vi "Cross Calibration.vi"(4 "RF data Out":T2={"Sampling Rate"=10, "Delay (micro s)"=0.08, "rf points per line"=3000} {"Delay (micro s)" format="%.2f"}, 6 "Vert Settings":cluster{u16, i32, "Coupling":u16}={4, 0, "Coupling"=2}, 8 "Motion Bd ID":T1=1 min=1 max=32 step=1) -> ()   [LabVIEW 2022 SP3]
uses:
  <instrlib>/Acqiris Dx/Acqiris Dx.lvlib
  ScanningControl/Motion Controllers/-MotionRoutines/MotionGlobals.vi
  <instrlib>/niScope/Acquire/Fetch/niScope Fetch.vi
  <vilib>/Utility/file.llb/Write To Spreadsheet File (string).vi
  <vilib>/Utility/file.llb/Write To Spreadsheet File (DBL).vi
  <vilib>/measure/NI_MAPro.lvlib
  <vilib>/measure/mascope.llb/Amplitude and Levels 1 chan.vi
  <vilib>/Math Plots/3D Math Plots/3D Surface/3D Surface Datatype/3D Surface Datatype.lvclass
  <vilib>/Math Plots/3D Math Plots/3D Surface/3D Surface Datatype/Public/Plot Helper (Vector).vi
  <vilib>/Analysis/NI_AALBase.lvlib
  <vilib>/Analysis/baseanly.llb/Mean (DBL).vi
  <vilib>/Math Plots/3D Math Plots/3D Surface/3D Surface XCtrl/3D Surface.xctl
panel:
  in  "Inverting Hydrophone?":bool
  in  "Main Digitizer":u16(ring)=1 items=["Acqiris Digitzer", "NI Digitizer"]
  in  "Notes":string="Tabor-DC Block-LPF-20dB attn- DC Block-ENI-Diode Expanders-PI50 ----- F22-06T-FOH System- Acqiris"
  in  "Amplifier Info":string="ENI 350L No Gauge"
  in  "Record Window (uS)":dbl=1.0
  in  "File Path":path=path "E:/Temp/PI50"
  in  "Auto Save Data?":bool
  out "Numeric":i32=8
  out "Numeric 2":i32=15
  in  "Save Waveforms":bool
  out "Waveform Array":dbl[][][](array[numeric])
  in  "Hydrophone Info":string="F22-06T"
  in  "Transducer Info":string(combo)="PI50-2-LPF-20dB"
  out "Ch 1":refnum<class "3D Plot Datatype.lvclass">[](xcontrol)
  out "Ch 0":refnum<class "3D Plot Datatype.lvclass">[](xcontrol)
  out "Ch 1":dbl[](graph)
  out "Ch 0":dbl[](graph)=[0.0, -0.000390625, -0.001953125, -0.0027343750000000003, -0.003125, -0.003125, -0.00390625, -0.004687500000000001, -0.005078125, -0.004687500000000001, -0.0027343750000000003, -0.00078125, 0.0015625, 0.0023437500000000003, 0.003515625, 0.004687500000000001, 0.005859375, 0.0054687500000000005, 0.004687500000000001, 0.00390625, 0.0027343750000000003, 0.000390625, -0.0027343750000000003, -0.004687500000000001, -0.005859375, -0.00625, -0.005859375, -0.00390625, -0.0023437500000000003, -0.000390625, 0.00078125, 0.0011718750000000002, 0.00078125, 0.0, -0.0015625, -0.0027343750000000003, -0.003515625, -0.00390625, -0.004296875, -0.0054687500000000005, -0.005859375, -0.0054687500000000005, -0.004687500000000001, -0.004296875, -0.00390625, -0.001953125, 0.00078125, 0.003515625, 0.003515625, 0.0027343750000000003, 0.00078125, -0.000390625, -0.0015625, -0.00078125, -0.00078125, -0.001953125, -0.00390625, -0.0054687500000000005, -0.00625, -0.005078125, -0.004687500000000001, -0.004296875, -0.003515625, -0.0015625, 0.000390625, 0.0015625, 0.0011718750000000002, 0.00078125, 0.0015625, 0.0027343750000000003, 0.0023437500000000003, 0.0, -0.0015625, -0.001953125, -0.00078125, -0.000390625, -0.000390625, 0.0, 0.000390625, 0.0011718750000000002, 0.0023437500000000003, 0.00390625, 0.004296875, 0.004687500000000001, 0.005078125, 0.005859375, 0.0054687500000000005, 0.004687500000000001, 0.003125, 0.001953125, 0.0, -0.001953125, -0.004296875, -0.00625, -0.00703125, -0.00703125, -0.004687500000000001, -0.003125, -0.0015625, -0.000390625, 0.000390625, 0.0, -0.0011718750000000002, -0.0027343750000000003, -0.004296875, -0.005078125, -0.005078125, -0.005859375, -0.00625, -0.006640625000000001, -0.00625, -0.00390625, -0.001953125, -0.0015625, -0.0011718750000000002, 0.0011718750000000002, 0.0023437500000000003, 0.003125, 0.003125, 0.003125, 0.003515625, 0.003125, 0.0027343750000000003, 0.0011718750000000002, -0.0015625, -0.003125, -0.003515625, -0.0011718750000000002, 0.0015625, 0.004687500000000001, 0.005859375, 0.0054687500000000005, 0.004296875, 0.003125, 0.0023437500000000003, 0.000390625, -0.0011718750000000002, -0.0023437500000000003, -0.003515625, -0.004687500000000001, -0.005078125, -0.005859375, -0.006640625000000001, -0.00703125, -0.0054687500000000005, -0.0027343750000000003, -0.000390625, 0.00078125, 0.0011718750000000002, 0.0015625, 0.0015625, 0.003515625, 0.003515625, 0.0015625, -0.00078125, -0.0015625, -0.001953125, -0.0015625, -0.0015625, -0.001953125, -0.001953125, -0.00078125, 0.00078125, 0.003125, 0.00390625, 0.00390625, 0.003125, 0.0027343750000000003, 0.0027343750000000003, 0.0023437500000000003, 0.0027343750000000003, 0.0011718750000000002, -0.00078125, -0.0027343750000000003, -0.0027343750000000003, -0.0023437500000000003, -0.0015625, -0.001953125, -0.003125, -0.003125, -0.0027343750000000003, -0.0011718750000000002, 0.0, 0.00078125, -0.00078125, -0.0015625, -0.0023437500000000003, -0.0027343750000000003, -0.00390625, -0.0054687500000000005, -0.005859375, -0.004687500000000001, -0.0027343750000000003, -0.0015625, -0.0015625, -0.000390625, -0.000390625, 0.00078125, 0.001953125, 0.0023437500000000003, 0.0027343750000000003, 0.0015625, 0.0, -0.0011718750000000002, -0.0015625, -0.001953125, -0.001953125, -0.001953125, -0.001953125, -0.00078125, -0.000390625, -0.000390625, 0.0, 0.0015625, 0.00390625, 0.0054687500000000005, 0.005859375, 0.0054687500000000005, 0.004687500000000001, 0.0027343750000000003, 0.00078125, -0.0011718750000000002, -0.003125, -0.0027343750000000003, -0.0027343750000000003, -0.0023437500000000003, -0.003515625, -0.003515625, -0.003515625, -0.0027343750000000003, -0.0015625, -0.00078125, -0.00078125, -0.0015625, -0.0023437500000000003, -0.0027343750000000003, -0.003515625, -0.00390625, -0.00390625, -0.005078125, -0.00703125, -0.0078125, -0.00703125, -0.0054687500000000005, -0.003125, -0.001953125, -0.00078125, 0.0, 0.000390625, 0.0, -0.0011718750000000002, -0.0023437500000000003, -0.00390625, -0.004687500000000001, -0.005078125, -0.005078125, -0.0054687500000000005, -0.006640625000000001, -0.006640625000000001, -0.00625, -0.004687500000000001, -0.003515625, -0.003515625, -0.003125, -0.0023437500000000003, -0.000390625, 0.0011718750000000002, 0.00078125, -0.000390625, -0.001953125, -0.0023437500000000003, -0.003125, -0.003515625, -0.00390625, -0.004687500000000001, -0.004296875, -0.003515625, -0.0023437500000000003, -0.000390625, 0.00078125, 0.001953125, 0.00390625, 0.005078125, 0.0054687500000000005, 0.00390625, 0.003515625, 0.0023437500000000003, 0.00078125, -0.0015625, -0.003125, -0.003125, -0.00390625, -0.004687500000000001, -0.0054687500000000005, -0.004687500000000001, -0.0027343750000000003, 0.0, 0.0023437500000000003, 0.003515625, 0.003515625, 0.00390625, 0.00390625, 0.003515625, 0.00078125, -0.0023437500000000003, -0.003125, -0.003125, -0.003125, -0.0023437500000000003, -0.0015625, -0.0011718750000000002, 0.0, 0.000390625, 0.0011718750000000002, 0.0015625, 0.0023437500000000003, 0.003125, 0.00390625, 0.003515625, 0.0023437500000000003, 0.00078125, -0.000390625, -0.001953125, -0.003125, -0.003125, -0.0027343750000000003, -0.0015625, -0.000390625, 0.0, 0.00078125, 0.0027343750000000003, 0.004296875, 0.004296875, 0.0023437500000000003, 0.0023437500000000003, 0.003515625, 0.005078125, 0.004687500000000001, 0.0023437500000000003, 0.0, -0.000390625, 0.0011718750000000002, 0.003125, 0.003125, 0.0015625, 0.000390625, 0.00078125, 0.0027343750000000003, 0.004687500000000001, 0.005859375, 0.004687500000000001, 0.003515625, 0.003125, 0.0027343750000000003, 0.003125, 0.0023437500000000003, 0.000390625, -0.00078125, -0.00078125, -0.000390625, 0.0, 0.0, 0.00078125, 0.0027343750000000003, 0.004687500000000001, 0.005078125, 0.004687500000000001, 0.004687500000000001, 0.005078125, 0.005078125, 0.003515625, 0.00078125, -0.0015625, -0.0015625, -0.0015625, -0.0015625, -0.00078125, -0.000390625, 0.000390625, 0.0011718750000000002, 0.0015625, 0.001953125, 0.0027343750000000003, 0.003515625, 0.00390625, 0.004296875, 0.00390625, 0.0023437500000000003, 0.000390625, -0.0011718750000000002, -0.0015625, -0.0023437500000000003, -0.0027343750000000003, -0.003125, -0.001953125, 0.00078125, 0.0027343750000000003, 0.004687500000000001, 0.0054687500000000005, 0.005859375, 0.005078125, 0.004296875, 0.003515625, 0.001953125, -0.000390625, -0.003125, -0.005078125, -0.00625, -0.006640625000000001, -0.00625, -0.005859375, -0.004296875, -0.003125, -0.0023437500000000003, -0.0015625, -0.000390625, 0.00078125, 0.0015625, 0.0015625, 0.0015625, 0.000390625, -0.0015625, -0.0023437500000000003, -0.0023437500000000003, -0.0023437500000000003, -0.001953125, -0.001953125, -0.0015625, -0.00078125, 0.0, 0.00078125, 0.0015625, 0.00078125, -0.000390625, -0.0023437500000000003, -0.0027343750000000003, -0.001953125, -0.0023437500000000003, -0.003515625, -0.004296875, -0.004687500000000001, -0.004296875, -0.004687500000000001, -0.005078125, -0.004687500000000001, -0.003125, -0.0015625, -0.00078125, -0.000390625, 0.000390625, 0.0011718750000000002, 0.001953125, 0.0015625, 0.0015625, 0.0015625, 0.0011718750000000002, 0.00078125, 0.000390625, -0.000390625, -0.0015625, -0.0011718750000000002, 0.000390625, 0.0015625, 0.0027343750000000003, 0.003515625, 0.004296875, 0.004296875, 0.004296875, 0.004296875, 0.004296875, 0.0027343750000000003, 0.0011718750000000002, -0.000390625, -0.0011718750000000002, -0.0015625, -0.001953125, -0.0015625, -0.00078125, 0.0, 0.0015625, 0.003125, 0.004296875, 0.0054687500000000005, 0.005859375, 0.00625, 0.00625, 0.005078125, 0.003125, 0.0011718750000000002, -0.00078125, -0.001953125, -0.003515625, -0.0054687500000000005, -0.006640625000000001, -0.006640625000000001, -0.005078125, -0.004296875, -0.0027343750000000003, -0.0023437500000000003, -0.00078125, 0.00078125, 0.001953125, 0.0011718750000000002, -0.00078125, -0.0023437500000000003, -0.0023437500000000003, -0.0015625, -0.00078125, -0.00078125, 0.0, 0.00078125, 0.001953125, 0.0023437500000000003, 0.0027343750000000003, 0.0023437500000000003, 0.001953125, 0.0023437500000000003, 0.003515625, 0.003515625, 0.0023437500000000003, 0.0011718750000000002, 0.000390625, 0.00078125, 0.00078125, -0.00078125, -0.003125, -0.003515625, -0.0027343750000000003, -0.0011718750000000002, -0.000390625, -0.0011718750000000002, -0.001953125, -0.0015625, 0.0, 0.00078125, 0.000390625, -0.00078125, -0.0011718750000000002, -0.00078125, -0.00078125, -0.001953125, -0.004687500000000001, -0.005859375, -0.004687500000000001, -0.0023437500000000003, -0.00078125, 0.000390625, 0.0023437500000000003, 0.00390625, 0.004296875, 0.003515625, 0.0023437500000000003, 0.0027343750000000003, 0.003125, 0.003125, 0.001953125, 0.0011718750000000002, 0.0, -0.000390625, 0.0, 0.0011718750000000002, 0.001953125, 0.003125, 0.004296875, 0.0054687500000000005, 0.005859375, 0.00625, 0.006640625000000001, 0.00703125, 0.0054687500000000005, 0.003515625, 0.0011718750000000002, -0.00078125, -0.0011718750000000002, -0.001953125, -0.0015625, -0.001953125, -0.0011718750000000002, 0.00078125, 0.0027343750000000003, 0.004296875, 0.004296875, 0.00390625, 0.00390625, 0.003125, 0.003125, 0.0011718750000000002, -0.0015625, -0.00390625, -0.004687500000000001, -0.004687500000000001, -0.004296875, -0.004296875, -0.00390625, -0.003125, -0.0015625, -0.000390625, 0.0, 0.0, -0.000390625, -0.000390625, -0.000390625, -0.00078125, -0.001953125, -0.003125, -0.003515625, -0.003515625, -0.003125, -0.003515625, -0.003125, -0.0023437500000000003, -0.00078125, 0.0011718750000000002, 0.003125, 0.004687500000000001, 0.005859375, 0.00703125, 0.0078125, 0.005859375, 0.004296875, 0.003125, 0.0015625, 0.000390625, 0.0, -0.000390625, -0.0011718750000000002, -0.001953125, -0.0015625, -0.000390625, 0.0011718750000000002, 0.0011718750000000002, 0.0, -0.0027343750000000003, -0.003515625, -0.0023437500000000003, -0.0015625, -0.0015625, -0.0023437500000000003, -0.0023437500000000003, -0.003125, -0.00390625, -0.004687500000000001, -0.004687500000000001, -0.00390625, -0.003515625, -0.0023437500000000003, -0.0015625, 0.0, 0.0015625, 0.0027343750000000003, 0.004296875, 0.004687500000000001, 0.003515625, 0.0023437500000000003, 0.0015625, 0.00078125, 0.0, -0.0015625, -0.0015625, -0.000390625, 0.000390625, 0.000390625, -0.000390625, -0.00078125, -0.000390625, 0.00078125, 0.0015625, 0.0015625, 0.0015625, 0.000390625, -0.00078125, -0.001953125, -0.003125, -0.004296875, -0.004687500000000001, -0.005078125, -0.004296875, -0.0023437500000000003, 0.0, 0.0015625, 0.003125, 0.005078125, 0.006640625000000001, 0.0074218750000000005, 0.008203125, 0.0074218750000000005, 0.006640625000000001, 0.00390625, 0.00078125, -0.0023437500000000003, -0.003125, -0.0023437500000000003, -0.0015625, 0.0, 0.000390625, 0.00078125, 0.001953125, 0.005859375, 0.008203125, 0.0078125, 0.005859375, 0.00390625, 0.0027343750000000003, 0.0015625, -0.00078125, -0.003515625, -0.004687500000000001, -0.004296875, -0.004296875, -0.003515625, -0.0027343750000000003, 0.0, 0.001953125, 0.004296875, 0.004687500000000001, 0.003125, 0.003515625, 0.00390625, 0.004296875, 0.00390625, 0.003515625, 0.003125, 0.001953125, 0.000390625, -0.00078125, -0.0011718750000000002, -0.0015625, -0.00078125, 0.000390625, 0.00078125, 0.0015625, 0.00078125, 0.0011718750000000002, 0.0015625, 0.0023437500000000003, 0.001953125, 0.00078125, -0.0015625, -0.003515625, -0.004687500000000001, -0.005078125, -0.00625, -0.0078125, -0.008203125, -0.00625, -0.001953125, 0.0011718750000000002, 0.0027343750000000003, 0.003515625, 0.00390625, 0.003515625, 0.0027343750000000003, 0.00078125, -0.00078125, -0.0023437500000000003, -0.004296875, -0.006640625000000001, -0.0078125, -0.0074218750000000005, -0.004687500000000001, -0.0015625, 0.00078125, 0.00078125, 0.00078125, 0.0011718750000000002, 0.0015625, 0.001953125, 0.0015625, 0.0011718750000000002, 0.000390625, -0.0015625, -0.003125, -0.004687500000000001, -0.005078125, -0.00390625, -0.00078125, 0.0015625, 0.003125, 0.003125, 0.003125, 0.004296875, 0.0054687500000000005, 0.006640625000000001, 0.00703125, 0.006640625000000001, 0.005078125, 0.003515625, 0.0015625, 0.0, -0.00078125, -0.00078125, 0.0, -0.00078125, -0.00078125, 0.0, 0.001953125, 0.003125, 0.00390625, 0.004687500000000001, 0.004296875, 0.0027343750000000003, 0.0, -0.0023437500000000003, -0.003515625, -0.00390625, -0.003125, -0.0027343750000000003, -0.0027343750000000003, -0.003125, -0.003125, -0.0027343750000000003, -0.0023437500000000003, -0.0023437500000000003, -0.0027343750000000003, -0.0023437500000000003, -0.0015625, -0.000390625, 0.000390625, 0.000390625, -0.000390625, -0.0015625, -0.0023437500000000003, -0.0015625, -0.000390625, 0.0, 0.00078125, 0.0023437500000000003, 0.004687500000000001, 0.005859375, 0.005859375, 0.004687500000000001, 0.004296875, 0.003515625, 0.0023437500000000003, 0.0015625, 0.000390625, -0.000390625, -0.0015625, -0.0023437500000000003, -0.003515625, -0.00390625, -0.0023437500000000003, -0.00078125, 0.00078125, 0.000390625, 0.000390625, 0.0011718750000000002, 0.003125, 0.004687500000000001, 0.005078125, 0.004296875, 0.00390625, 0.004296875, 0.00390625, 0.0027343750000000003, 0.0015625, 0.00078125, 0.0, -0.00078125, -0.00078125, 0.000390625, 0.0015625, 0.003125, 0.004296875, 0.004687500000000001, 0.005078125, 0.00625, 0.006640625000000001, 0.0054687500000000005, 0.004296875, 0.0023437500000000003, 0.001953125, 0.001953125, 0.0027343750000000003, 0.001953125, 0.0, -0.0015625, -0.001953125, -0.0015625, -0.000390625, 0.00078125, 0.0011718750000000002, 0.0011718750000000002, -0.000390625, -0.0015625, -0.0027343750000000003, -0.0023437500000000003, -0.001953125, -0.0015625, -0.001953125, -0.003125, -0.00390625, -0.004296875, -0.004296875, -0.003125, -0.0015625, -0.000390625, 0.00078125, 0.003125, 0.005859375, 0.00703125, 0.00703125, 0.004687500000000001, 0.003125, 0.0015625, 0.000390625, -0.000390625, -0.000390625, -0.000390625, 0.0, 0.0011718750000000002, 0.0027343750000000003, 0.003515625, 0.00390625, 0.00390625, 0.004296875, 0.004687500000000001, 0.005078125, 0.0054687500000000005, 0.0054687500000000005, 0.004687500000000001, 0.003125, 0.0, -0.0023437500000000003, -0.001953125, 0.000390625, 0.0023437500000000003, 0.0023437500000000003, 0.0015625, 0.0011718750000000002, 0.0023437500000000003, 0.004687500000000001, 0.004687500000000001, 0.003515625, 0.0011718750000000002, -0.000390625, -0.00078125, 0.000390625, -0.00078125, -0.00390625, -0.00625, -0.006640625000000001, -0.006640625000000001, -0.005859375, -0.0054687500000000005, -0.004687500000000001, -0.003125, -0.000390625, 0.0023437500000000003, 0.00390625, 0.003125, 0.000390625, -0.0023437500000000003, -0.004687500000000001, -0.00390625, -0.0054687500000000005, -0.0078125, -0.008984375000000001, -0.00703125, -0.004296875, -0.0011718750000000002, 0.0015625, 0.0023437500000000003, 0.0027343750000000003, 0.004296875, 0.005859375, 0.006640625000000001, 0.005859375, 0.003515625, 0.0015625, 0.00078125, -0.000390625, -0.0015625, -0.0015625, -0.00078125, 0.000390625, 0.000390625, 0.0011718750000000002, 0.0023437500000000003, 0.003125, 0.00390625, 0.004296875, 0.00390625, 0.004296875, 0.004687500000000001, 0.003515625, 0.0023437500000000003, 0.0015625, 0.001953125, 0.001953125, 0.001953125, 0.0027343750000000003, 0.0023437500000000003, 0.0015625, 0.000390625, -0.0011718750000000002, 0.0, 0.0015625, 0.0027343750000000003, 0.004296875]
  out "Data Array":cluster{dbl[], dbl[], dbl[], dbl[]}={[30.0, 30.0, 30.0, 30.0, 30.0, 30.0, 30.0, 30.0, 30.0, 32.0, 32.0, 32.0, 32.0, 32.0, 32.0, 32.0, 32.0, 32.0, 34.0, 34.0, 34.0, 34.0, 34.0, 34.0, 34.0, 34.0, 34.0, 36.0, 36.0, 36.0, 36.0, 36.0, 36.0, 36.0, 36.0, 36.0, 38.0, 38.0, 38.0, 38.0, 38.0, 38.0, 38.0, 38.0, 38.0, 40.0, 40.0, 40.0, 40.0, 40.0, 40.0, 40.0, 40.0, 40.0, 42.0, 42.0, 42.0, 42.0, 42.0, 42.0, 42.0, 42.0, 42.0, 44.0, 44.0, 44.0, 44.0, 44.0, 44.0, 44.0, 44.0, 44.0, 46.0, 46.0, 46.0, 46.0, 46.0, 46.0, 46.0, 46.0, 46.0, 48.0, 48.0, 48.0, 48.0, 48.0, 48.0, 48.0, 48.0, 48.0, 50.0, 50.0, 50.0, 50.0, 50.0, 50.0, 50.0, 50.0, 50.0, 52.0, 52.0, 52.0, 52.0, 52.0, 52.0, 52.0, 52.0, 52.0, 54.0, 54.0, 54.0, 54.0, 54.0, 54.0, 54.0, 54.0, 54.0, 56.0, 56.0, 56.0, 56.0, 56.0, 56.0, 56.0, 56.0, 56.0, 58.0, 58.0, 58.0, 58.0, 58.0, 58.0, 58.0, 58.0, 58.0, 60.0, 60.0, 60.0, 60.0, 60.0, 60.0, 60.0, 60.0, 60.0], [0.1, 0.2, 0.30000000000000004, 0.4, 0.5, 0.6, 0.7000000000000001, 0.8, 0.9, 0.1, 0.2, 0.30000000000000004, 0.4, 0.5, 0.6, 0.7000000000000001, 0.8, 0.9, 0.1, 0.2, 0.30000000000000004, 0.4, 0.5, 0.6, 0.7000000000000001, 0.8, 0.9, 0.1, 0.2, 0.30000000000000004, 0.4, 0.5, 0.6, 0.7000000000000001, 0.8, 0.9, 0.1, 0.2, 0.30000000000000004, 0.4, 0.5, 0.6, 0.7000000000000001, 0.8, 0.9, 0.1, 0.2, 0.30000000000000004, 0.4, 0.5, 0.6, 0.7000000000000001, 0.8, 0.9, 0.1, 0.2, 0.30000000000000004, 0.4, 0.5, 0.6, 0.7000000000000001, 0.8, 0.9, 0.1, 0.2, 0.30000000000000004, 0.4, 0.5, 0.6, 0.7000000000000001, 0.8, 0.9, 0.1, 0.2, 0.30000000000000004, 0.4, 0.5, 0.6, 0.7000000000000001, 0.8, 0.9, 0.1, 0.2, 0.30000000000000004, 0.4, 0.5, 0.6, 0.7000000000000001, 0.8, 0.9, 0.1, 0.2, 0.30000000000000004, 0.4, 0.5, 0.6, 0.7000000000000001, 0.8, 0.9, 0.1, 0.2, 0.30000000000000004, 0.4, 0.5, 0.6, 0.7000000000000001, 0.8, 0.9, 0.1, 0.2, 0.30000000000000004, 0.4, 0.5, 0.6, 0.7000000000000001, 0.8, 0.9, 0.1, 0.2, 0.30000000000000004, 0.4, 0.5, 0.6, 0.7000000000000001, 0.8, 0.9, 0.1, 0.2, 0.30000000000000004, 0.4, 0.5, 0.6, 0.7000000000000001, 0.8, 0.9, 0.1, 0.2, 0.30000000000000004, 0.4, 0.5, 0.6, 0.7000000000000001, 0.8, 0.9], [0.004632148742675781, 0.012890625000000001, 0.02666015625, 0.040019531250000004, 0.05185546875, 0.059953498840332034, 0.06650390625, 0.07060546875, 0.0755859375, 0.004534759521484375, 0.012421875, 0.023457031250000003, 0.03400390625, 0.04359375, 0.05009765625, 0.05556640625, 0.059375, 0.063671875, 0.004769134521484375, 0.0134765625, 0.0256640625, 0.0360546875, 0.0433203125, 0.0474609375, 0.050820312500000006, 0.055703125000000006, 0.05859375, 0.005977287292480469, 0.014921875000000001, 0.02759765625, 0.03814453125, 0.04376953125, 0.0478515625, 0.052109375000000006, 0.0555859375, 0.0589453125, 0.005100135803222656, 0.01326171875, 0.02373046875, 0.0325, 0.0365234375, 0.039628906250000005, 0.04396484375, 0.046484375, 0.0507421875, 0.00481048583984375, 0.01208984375, 0.021328125000000003, 0.027714843750000002, 0.031542968750000004, 0.03357421875, 0.03666015625, 0.03853515625, 0.0409375, 0.0033821487426757813, 0.01138671875, 0.020722656250000002, 0.027246093750000002, 0.030507812500000002, 0.032207031250000004, 0.034824218750000004, 0.0376953125, 0.040156250000000004, 0.004744377136230469, 0.01, 0.01712890625, 0.020546875000000003, 0.02255859375, 0.024492187500000002, 0.025859375, 0.02880859375, 0.03125, 0.0044387817382812505, 0.008104858398437501, 0.01357421875, 0.015234375000000001, 0.01677734375, 0.01775390625, 0.0185546875, 0.019765625000000002, 0.021386718750000002, 0.004646453857421875, 0.007614898681640625, 0.0123828125, 0.014179687500000001, 0.01564453125, 0.0164453125, 0.017304687500000002, 0.0184765625, 0.0194921875, 0.00439453125, 0.0068927001953125, 0.011093750000000001, 0.01208984375, 0.01306640625, 0.01447265625, 0.015156250000000001, 0.0165234375, 0.01755859375, 0.00494110107421875, 0.004515190124511719, 0.010703125, 0.011484375, 0.01228515625, 0.0132421875, 0.01412109375, 0.015078125000000001, 0.016015625000000002, 0.003555717468261719, 0.006270446777343751, 0.00998046875, 0.01072265625, 0.01130859375, 0.012226562500000001, 0.01244140625, 0.0132421875, 0.014140625, 0.004312858581542969, 0.005177078247070313, 0.008241539001464845, 0.00966796875, 0.009765625, 0.010683593750000001, 0.011582031250000001, 0.012226562500000001, 0.0127734375, 0.004861183166503906, 0.005276260375976563, 0.007224807739257813, 0.006856727600097656, 0.008536224365234376, 0.008964920043945314, 0.010195312500000001, 0.010371093750000001, 0.0107421875, 0.005235977172851563, 0.004944725036621094, 0.00478424072265625, 0.0060133361816406255, 0.006972541809082032, 0.007910881042480469, 0.00812469482421875, 0.008906250000000001, 0.008612861633300781], [0.0, 0.0, 0.0, 0.0, 0.0, 0.0, 0.0, 0.0, 0.0, 0.0, 0.0, 0.0, 0.0, 0.0, 0.0, 0.0, 0.0, 0.0, 0.0, 0.0, 0.0, 0.0, 0.0, 0.0, 0.0, 0.0, 0.0, 0.0, 0.0, 0.0, 0.0, 0.0, 0.0, 0.0, 0.0, 0.0, 0.0, 0.0, 0.0, 0.0, 0.0, 0.0, 0.0, 0.0, 0.0, 0.0, 0.0, 0.0, 0.0, 0.0, 0.0, 0.0, 0.0, 0.0, 0.0, 0.0, 0.0, 0.0, 0.0, 0.0, 0.0, 0.0, 0.0, 0.0, 0.0, 0.0, 0.0, 0.0, 0.0, 0.0, 0.0, 0.0, 0.0, 0.0, 0.0, 0.0, 0.0, 0.0, 0.0, 0.0, 0.0, 0.0, 0.0, 0.0, 0.0, 0.0, 0.0, 0.0, 0.0, 0.0, 0.0, 0.0, 0.0, 0.0, 0.0, 0.0, 0.0, 0.0, 0.0, 0.0, 0.0, 0.0, 0.0, 0.0, 0.0, 0.0, 0.0, 0.0, 0.0, 0.0, 0.0, 0.0, 0.0, 0.0, 0.0, 0.0, 0.0, 0.0, 0.0, 0.0, 0.0, 0.0, 0.0, 0.0, 0.0, 0.0, 0.0, 0.0, 0.0, 0.0, 0.0, 0.0, 0.0, 0.0, 0.0, 0.0, 0.0, 0.0, 0.0, 0.0, 0.0, 0.0, 0.0, 0.0]}
  in  "Attenuator":dbl=1.0
  in  "Num Voltage Steps":i32=9
  in  "Average":i32=20
  out "current f":dbl=60.0
  in  "Freq Step Size (MHz)":dbl=2.0 format="%.2f"
  in  "Start frequency (MHz)":dbl=30.0 format="%.2f"
  in  "Cal Tran":bool
  in  "Set up Digi":bool
  in  "ExitSendCmd":bool
  in  "Save":bool
  out "current V":dbl=0.9
  in  "Function Generator":u16(ring)=1 items=["Agilent", "Tabor"]
  in  "Voltage Step Size (mVpp)":dbl=100.0 format="%.2f"
  in  "Num Freq Steps":i32=16
  in  "Start voltage (mVpp)":dbl=100.0 format="%.3f"
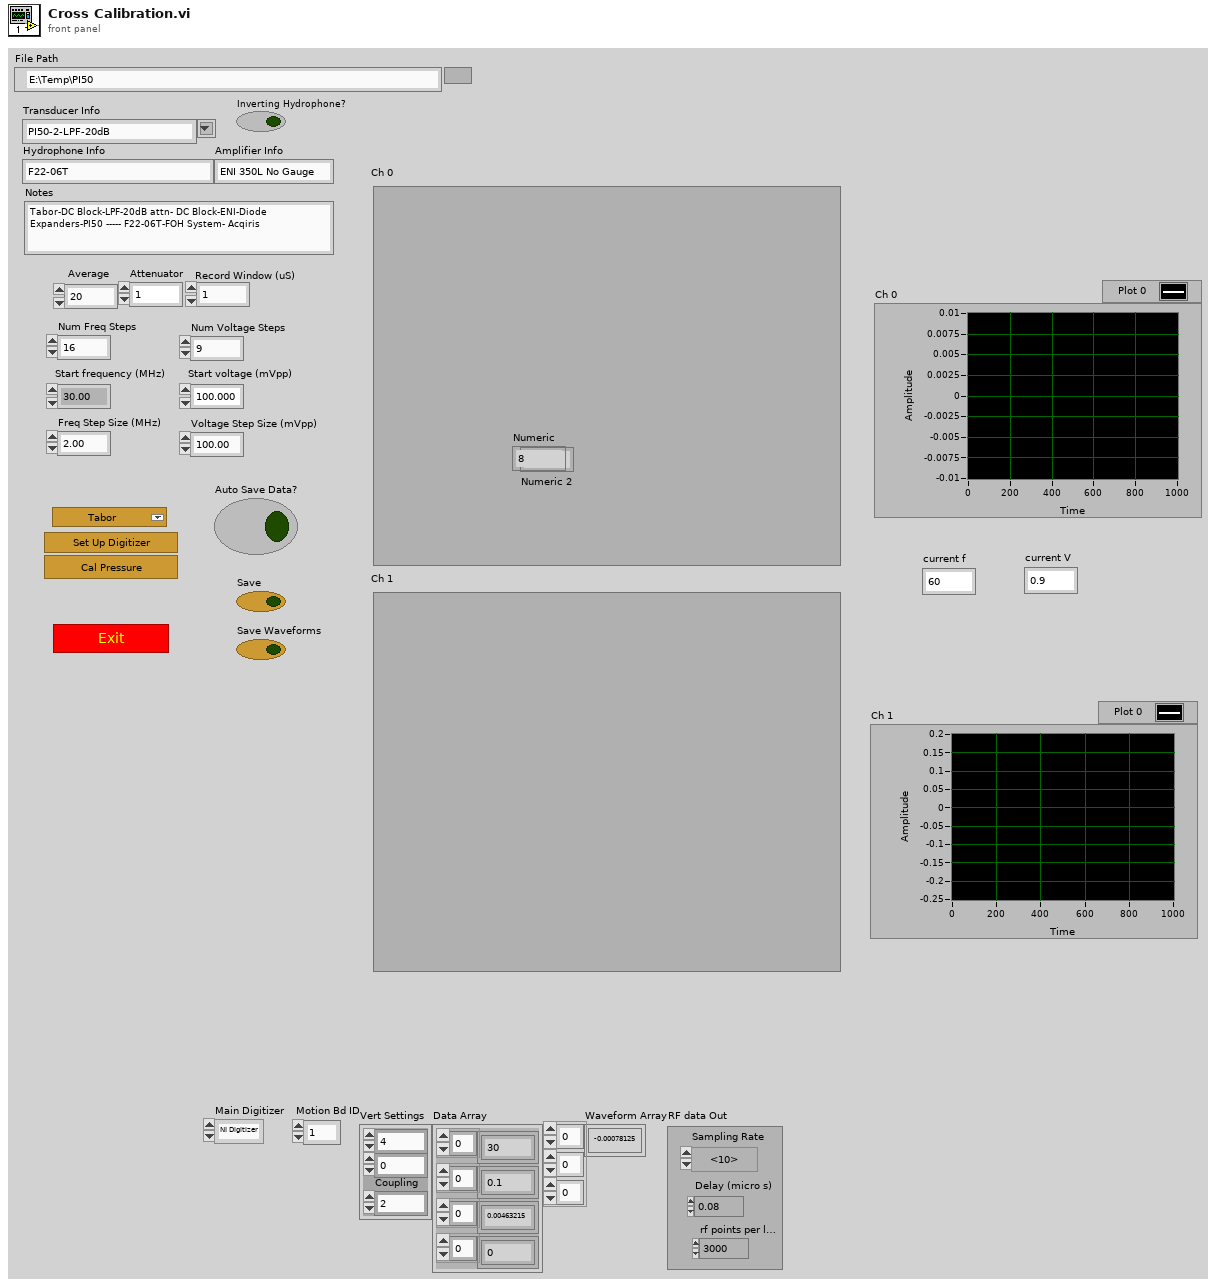
[diagram p1: front panel]
types:
  T1 = typedef "Board Id" = u8
  T2 = cluster{"Sampling Rate":u16, "Delay (micro s)":dbl, "rf points per line":u16}
  T3 = cluster{"Sampling Rate":dbl, "Ref Delay (ms)":dbl, "rf points per line":i32}
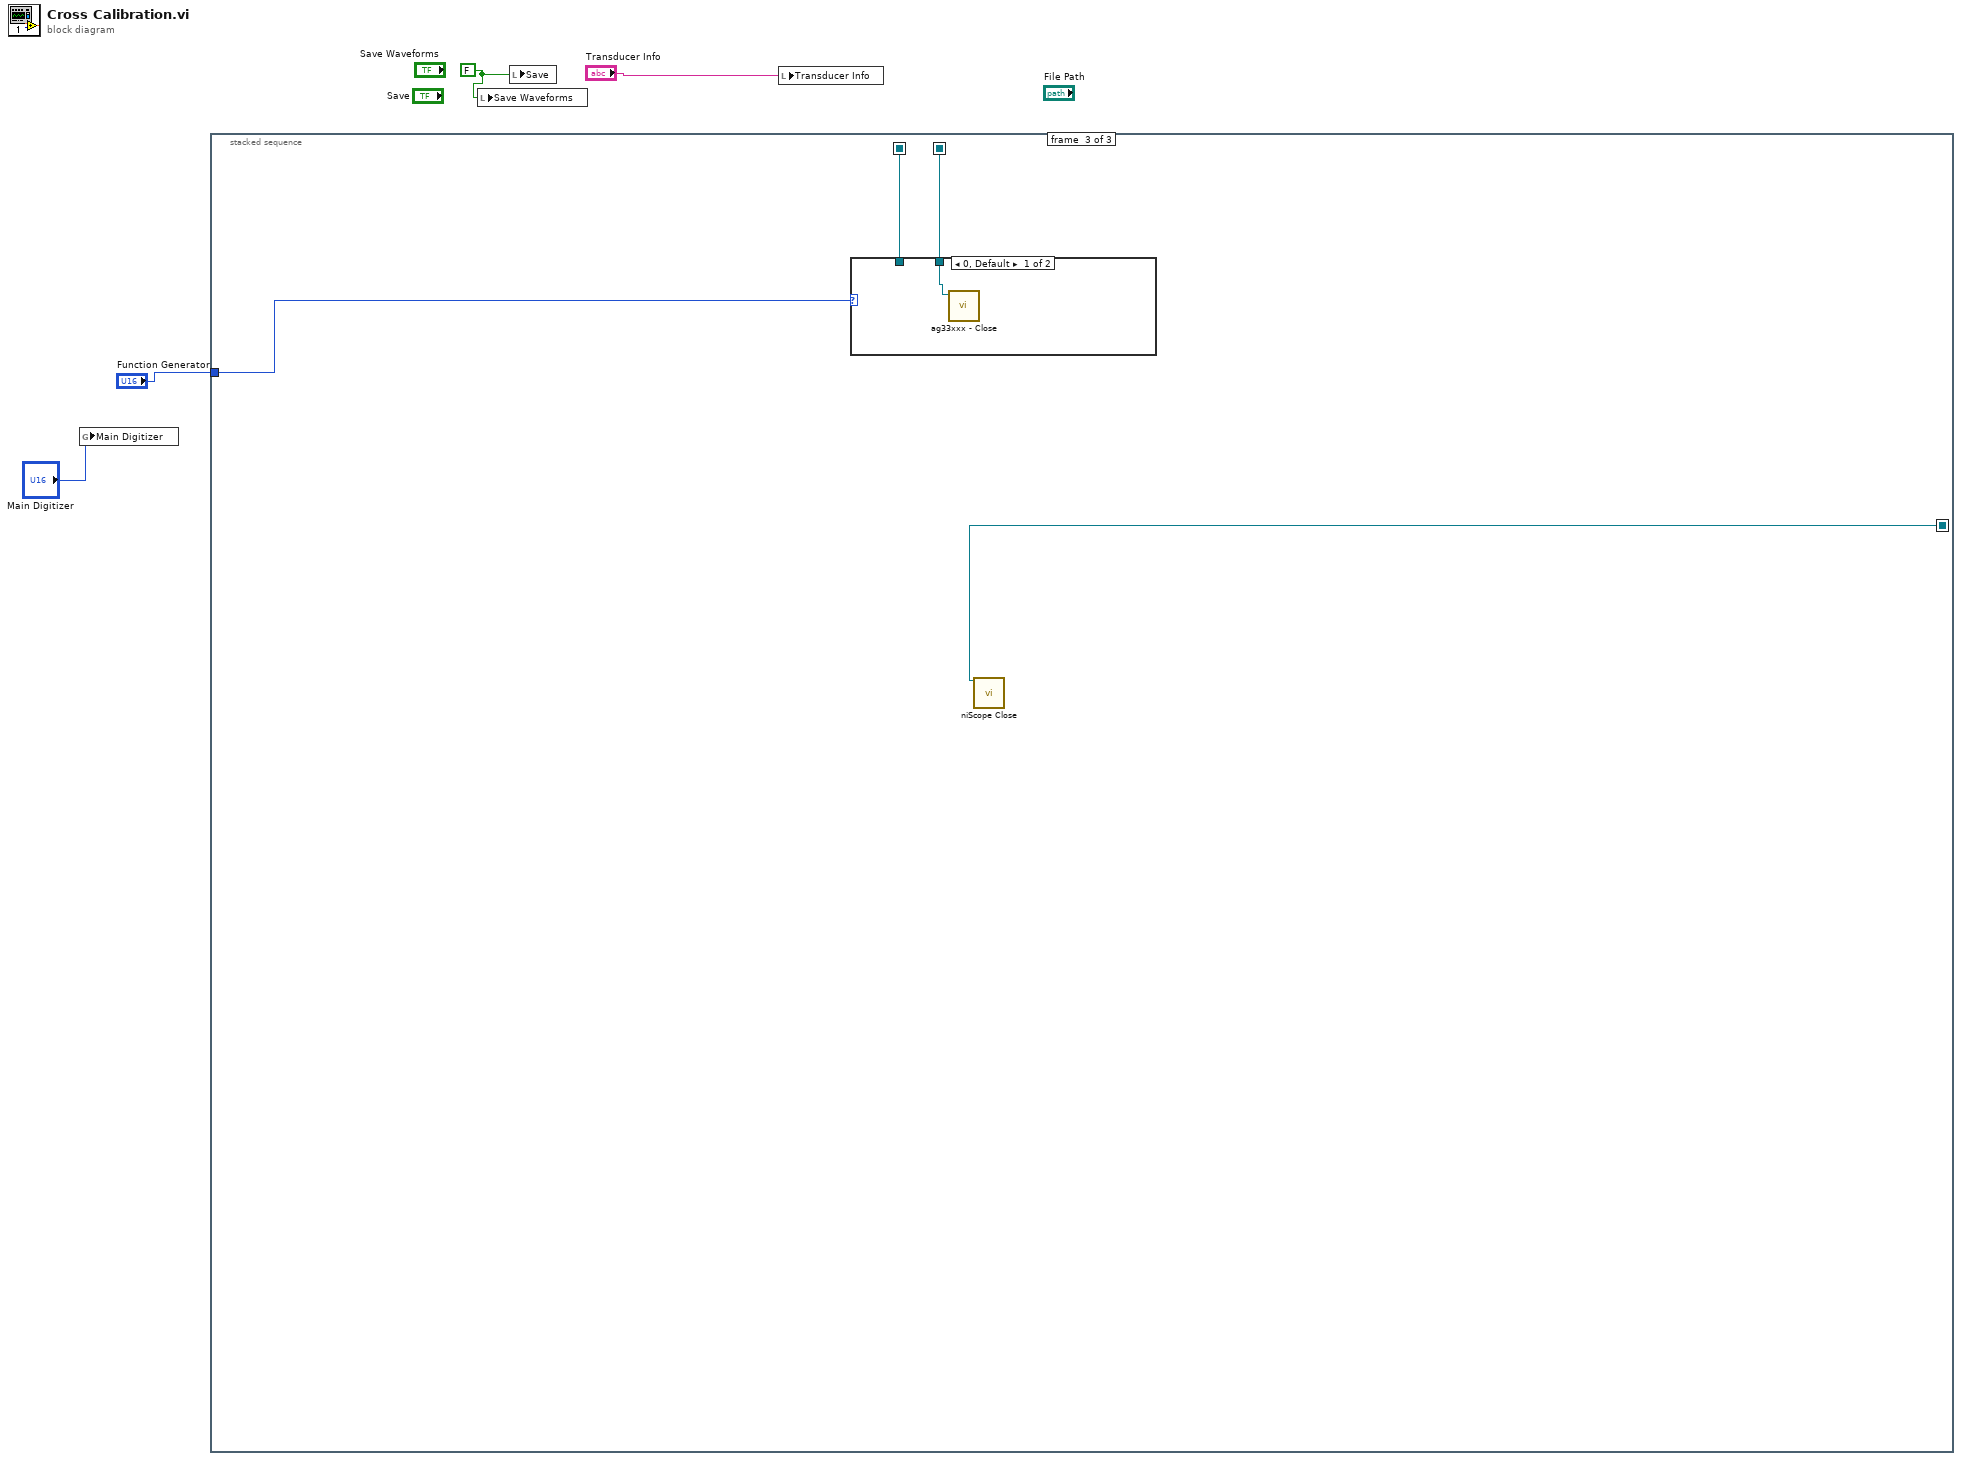
[diagram p0: block diagram]
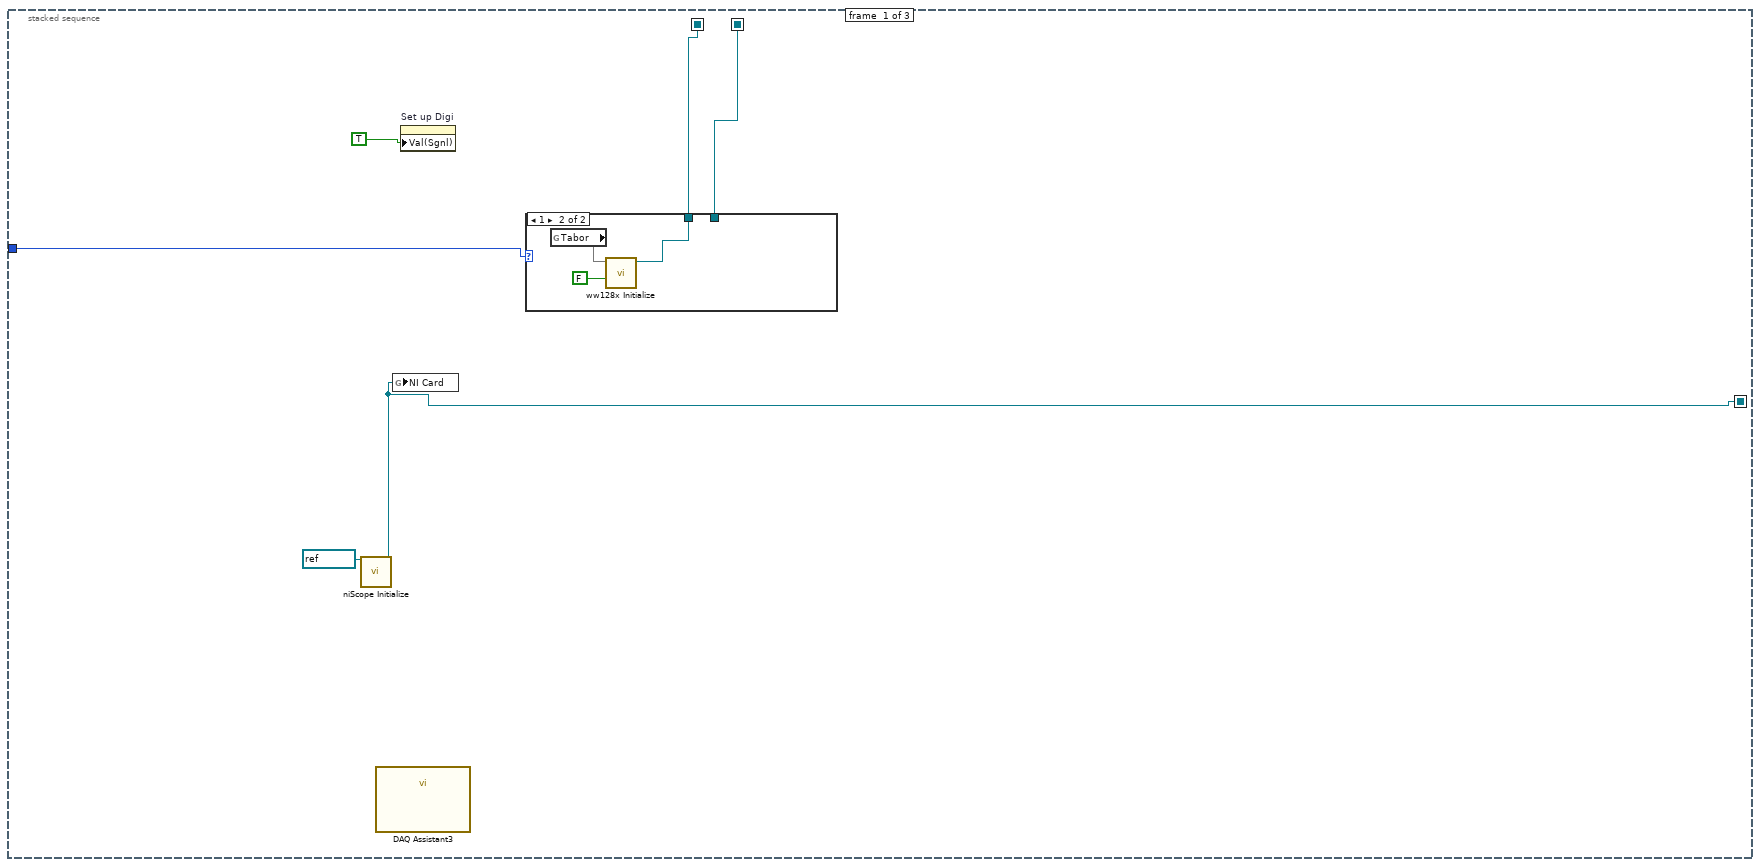
[diagram p2: hidden frame]
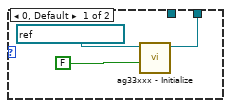
[diagram p3: hidden frame]
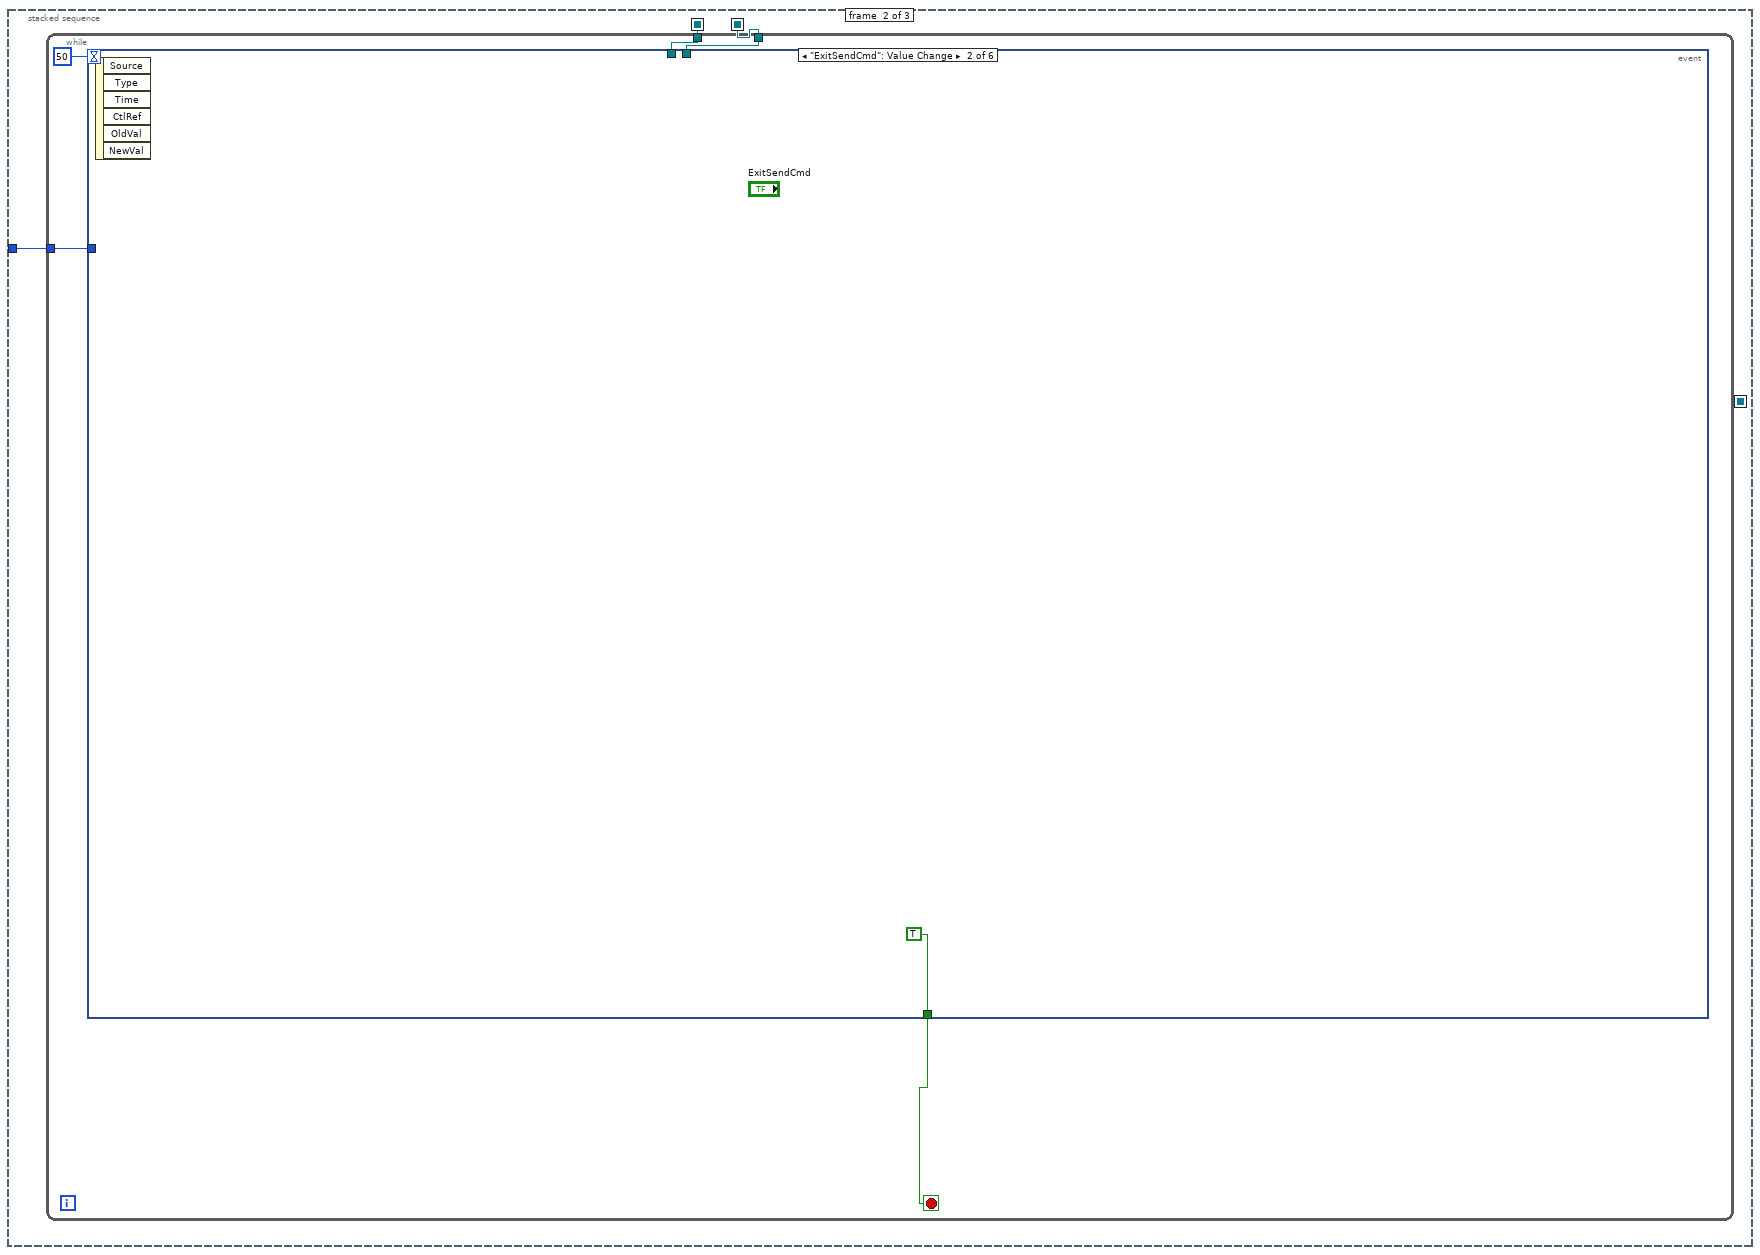
[diagram p4: hidden frame]
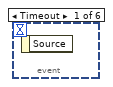
[diagram p5: hidden frame]
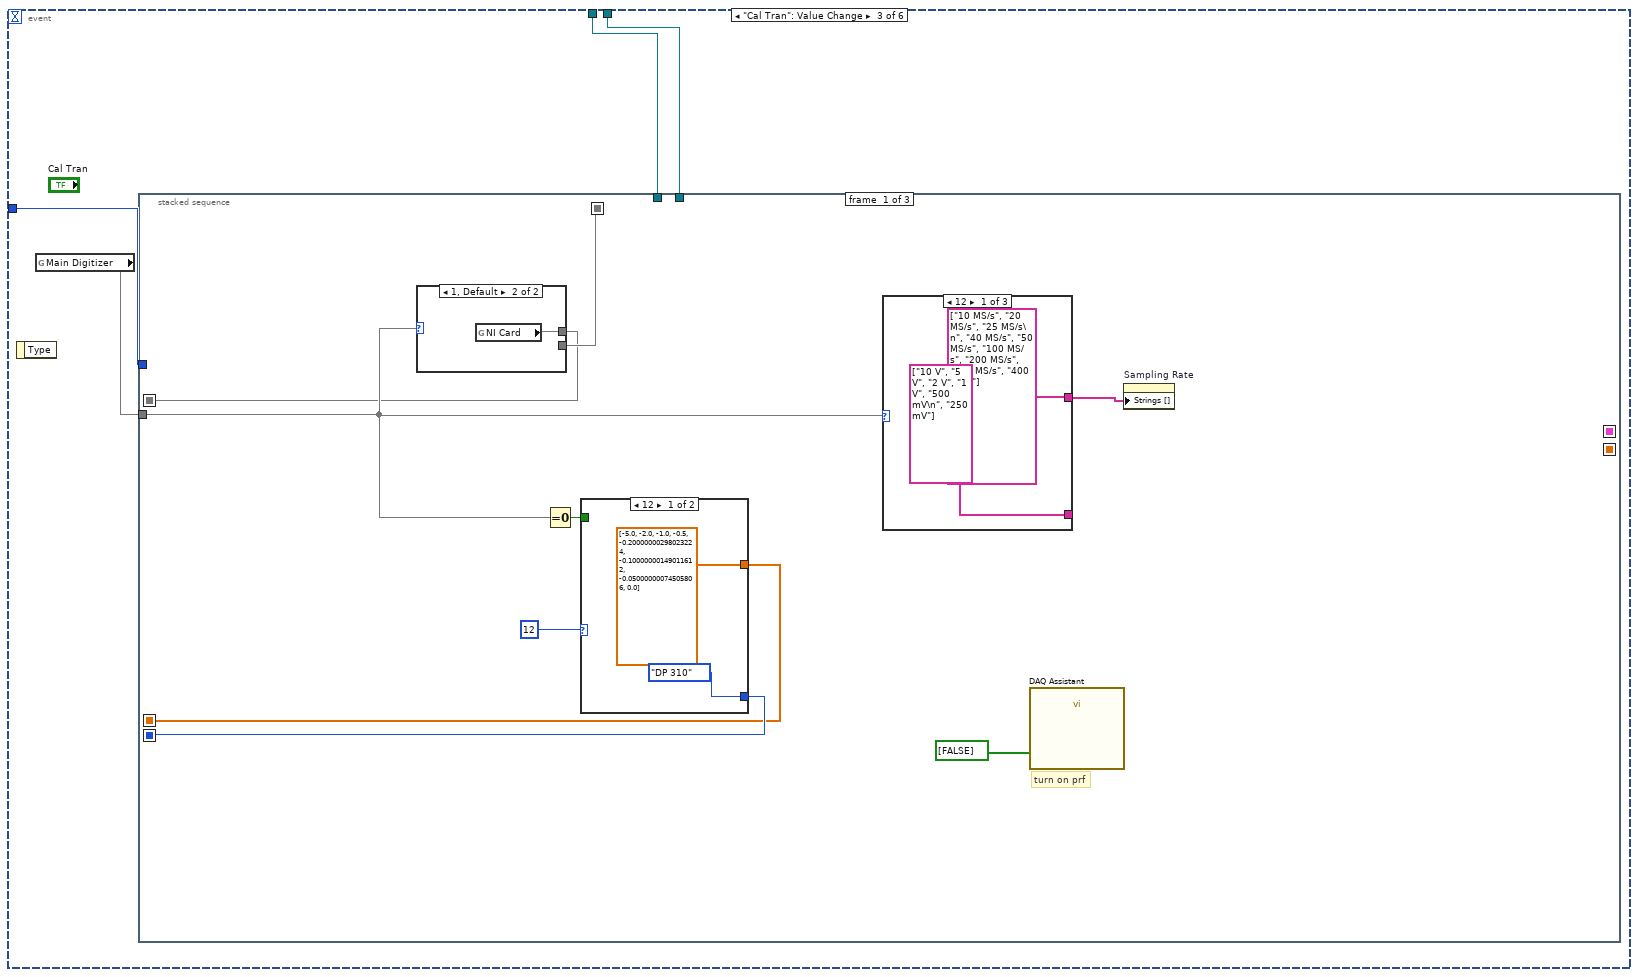
[diagram p6: hidden frame]
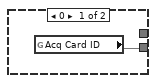
[diagram p7: hidden frame]
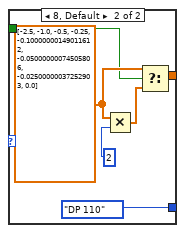
[diagram p8: hidden frame]
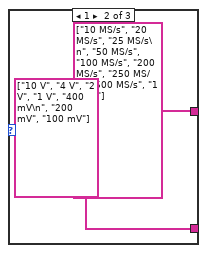
[diagram p9: hidden frame]
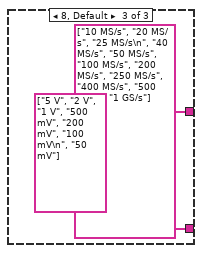
[diagram p10: hidden frame]
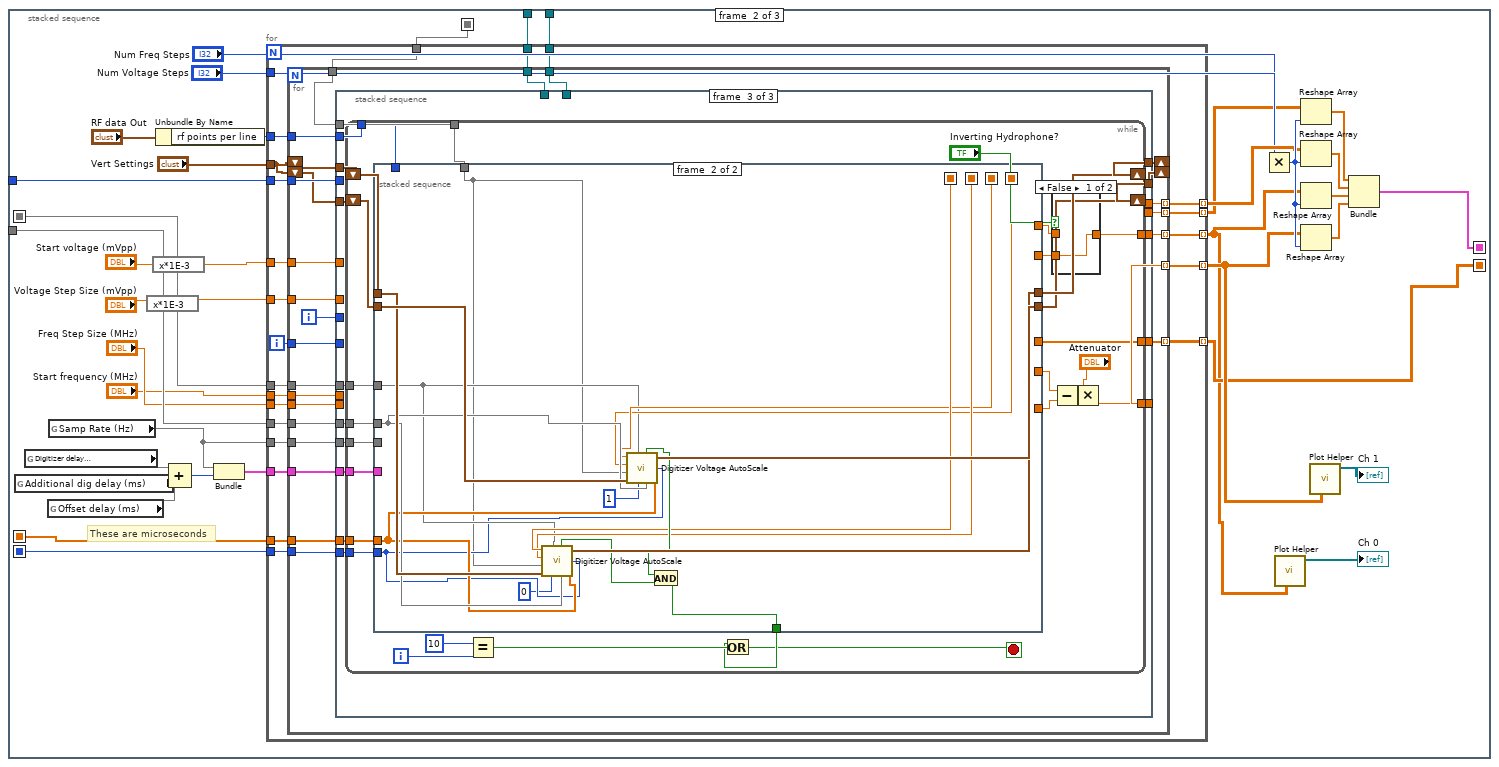
[diagram p11: hidden frame]
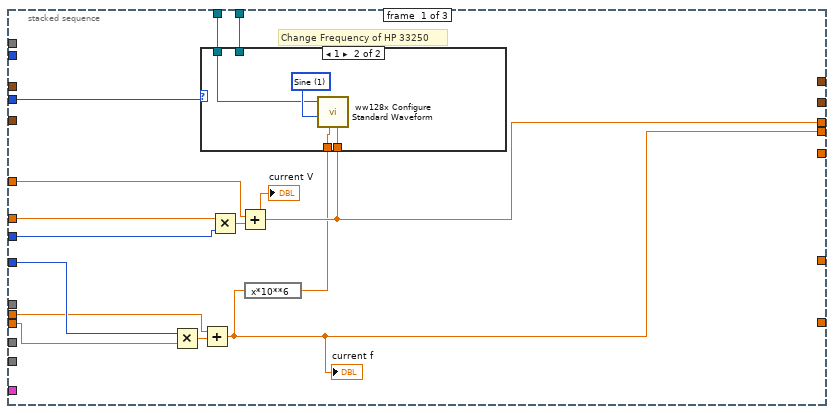
[diagram p12: hidden frame]
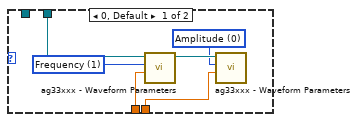
[diagram p13: hidden frame]
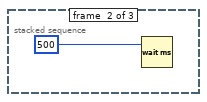
[diagram p14: hidden frame]
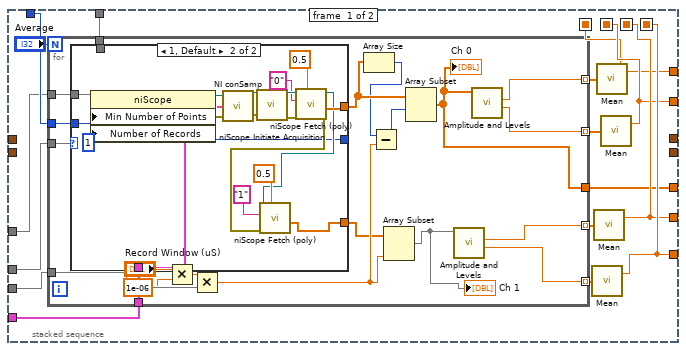
[diagram p16: hidden frame]
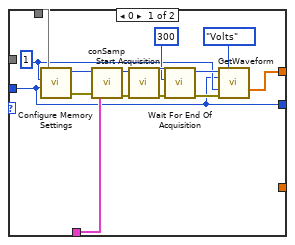
[diagram p17: hidden frame]
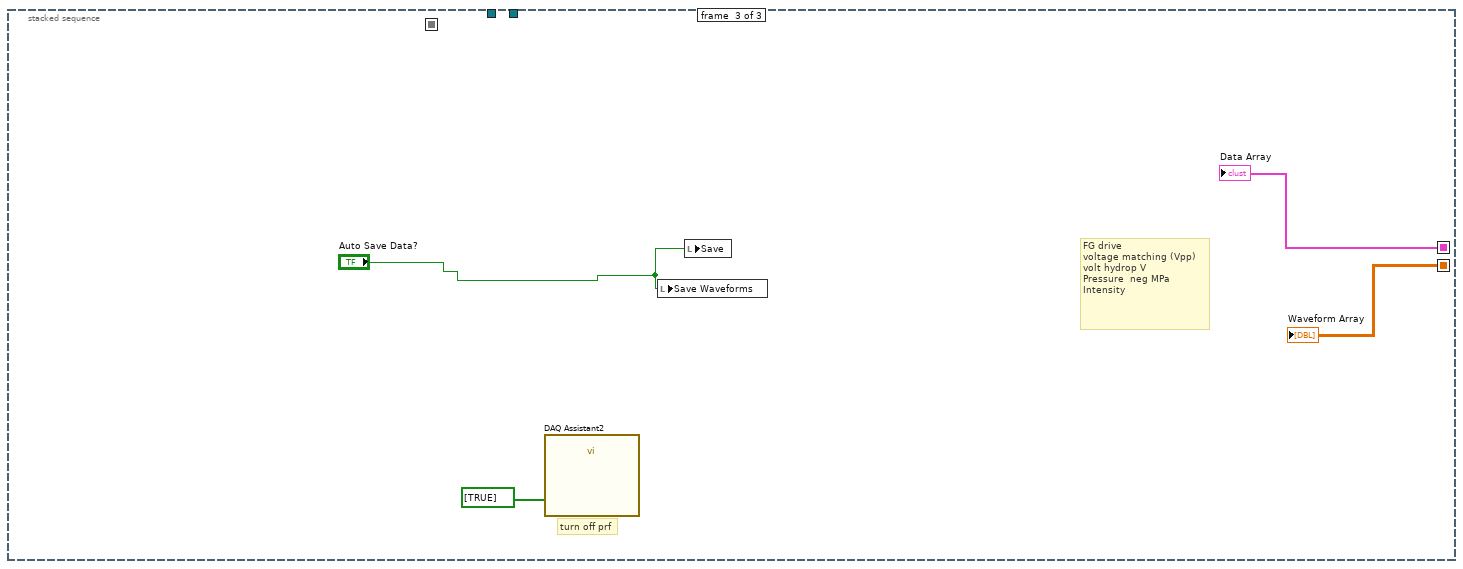
[diagram p18: hidden frame]
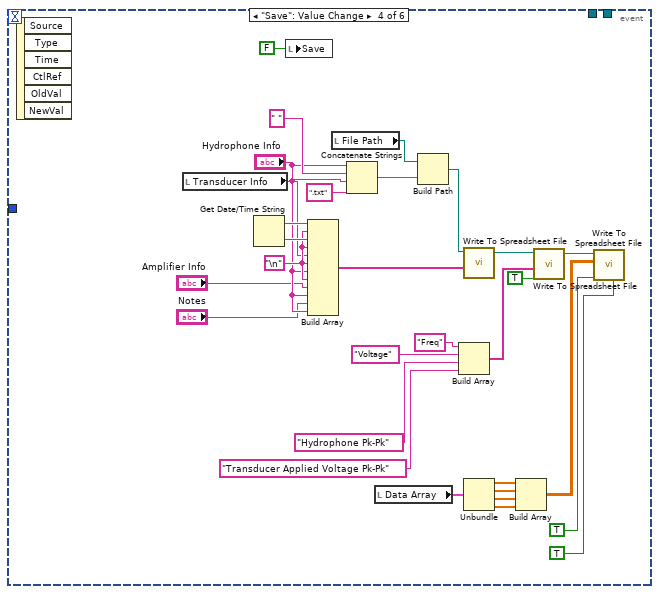
[diagram p19: hidden frame]
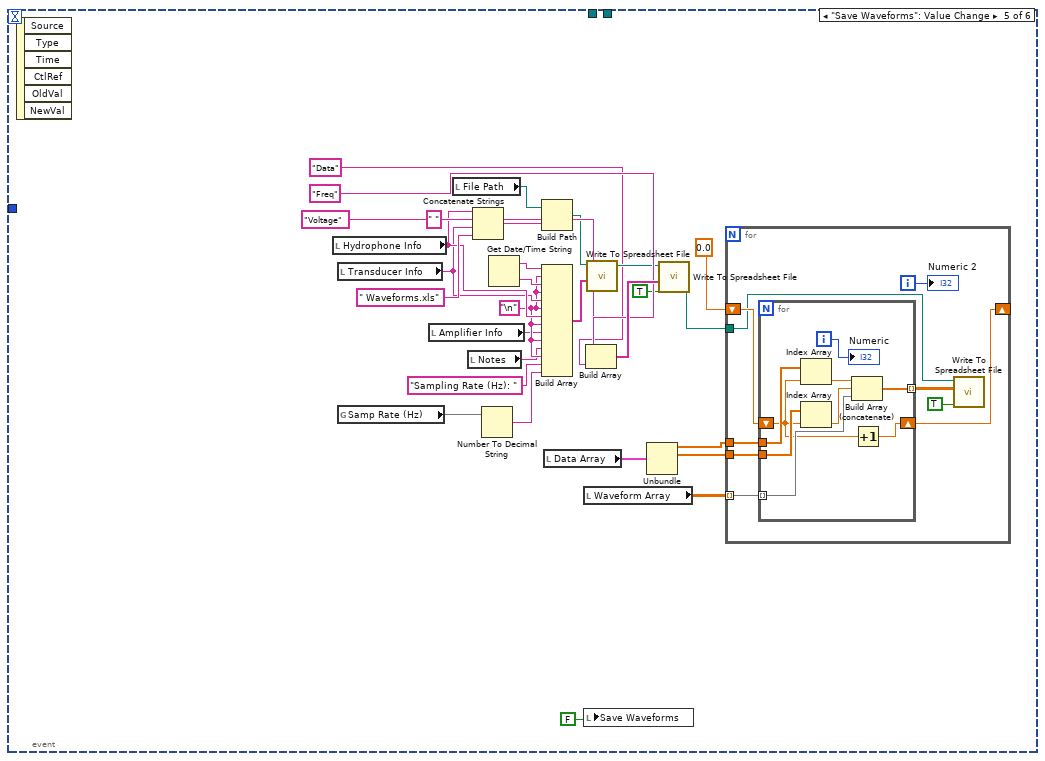
[diagram p20: hidden frame]
diagram:
  w1 = FALSE
  n1 = global write "MotionGlobals.vi" "Main Digitizer"("Main Digitizer") -> ()
  n2 = stacked-sequence {
    seq-local: [w8 _ _] -> [_ _ w388]
    seq-local: [w6 _ _] -> [_ w18 w386]
    seq-local: [w7 _ _] -> [_ w17 w385]
    tunnel: "Function Generator" -> [w9 w19 w387]
    frame #0 {
      n3 = call <instrlib>:"niScope Initialize.vi"("resource name"=refnum<k15> "DIG1") -> ("instrument handle"=w8:refnum<k15>)  [unwired: 3 in, 11 out]
      n4 = call "DAQ Assistant3"() -> ()  [unwired: 17 in, 3 out]
      n5 = global write "MotionGlobals.vi" "NI Card"(w8) -> ()
      n6 = property on="Set up Digi" class="Bool (strict)"("Val(Sgnl)"=TRUE) -> ()  [unwired: 2 in, 2 out]
      n7 = case shown="1" w9 {
        tunnel: [w12 _] -> w7
        tunnel: [_ w15] -> w6
        frame 0, Default {
          n8 = call <instrlib>:"ag33xxx - Initialize.vi"("Reset (T: Reset)"=FALSE, "Instrument Resource Name"=refnum<visa-resource-name> "GPIB::13::INSTR") -> ("dup VISA session"=w12:refnum<visa-resource-name>)  [unwired: 8 in, 1 out]
        }
        frame 1 {
          n9 = global read "MotionGlobals.vi" "Tabor"() -> (w14)
          n10 = call <instrlib>:"ww128x Initialize.vi"("reset device (Yes)"=FALSE ("reset device"), "resource name"=w14) -> ("instrument handle out"=w15:refnum<k15>)  [unwired: 2 in, 7 out]
        }
      }
    }
    frame #1 {
      n11 = while {
        tunnel: w19 -> [w22]
        tunnel: w18 -> [w21]
        tunnel: w17 -> [w20]
        stop <- w24 stop-if-true
        n12 = event shown="[1] \"ExitSendCmd\": Value Change" {
          selector: _ -> [_ _ _ _ _ _]
          dyn-events: _ -> [_ _ _ _ _ _]
          timeout: 50 -> [_ _ _ _ _ _]
          tunnel: [_ TRUE _ _ _ _] -> w24
          tunnel: w22 -> [_ _ w28 _ _ _]
          tunnel: w21 -> [_ _ w27 _ _ _]
          tunnel: w20 -> [_ _ w26 _ _ _]
          event Timeout {
            n13 = event-data() -> ()  [unwired: 2 out]
          }
          event "ExitSendCmd": Value Change {
            n14 = event-data() -> ()  [unwired: 7 out]
          }
          event "Cal Tran": Value Change {
            n15 = event-data() -> ()  [unwired: 2 out]
            n16 = global read "MotionGlobals.vi" "Main Digitizer"() -> (w29)
            n17 = stacked-sequence {
              seq-local: [w36 _ _] -> [_ w90 _]
              seq-local: [w37 _ _] -> [_ w91 _]
              seq-local: [w33 _ _] -> [_ w85 _]
              seq-local: [_ w76 _] -> [_ _ w300]
              seq-local: [w32 _ _] -> [_ w75 _]
              seq-local: [_ w57 _] -> [_ _ w299]
              tunnel: w29 -> [w35 w84 _]
              tunnel: w28 -> [_ w74 _]
              tunnel: w27 -> [_ w73 _]
              tunnel: w26 -> [_ w72 _]
              frame #0 {
                # "turn on prf"
                n18 = case shown="1, Default" w35 {
                  tunnel: [w39 _] -> w33
                  tunnel: [_ w40] -> w32
                  frame 0 {
                    n19 = global read "MotionGlobals.vi" "Acq Card ID"() -> (w39)
                  }
                  frame 1, Default {
                    n20 = global read "MotionGlobals.vi" "NI Card"() -> (w40)
                  }
                }
                n21 = Equal To 0?(x=w35) -> (x = 0?=w38:bool)
                n22 = case shown="12" 12 {
                  tunnel: [sgl[] [-5.0, -2.0, -1.0, -0.5, -0.2, -0.1, -0.05, 0.0] w43] -> w36
                  tunnel: [enum16{"DP 110", "DP 310"}."DP 310" ("Card Type") enum16{"DP 110", "DP 310"}."DP 110" ("Card Type")] -> w37
                  tunnel: w38 -> [_ w44]
                  frame 12 {
                  }
                  frame 8, Default {
                    w45 = sgl[] [-2.5, -1.0, -0.5, -0.25, -0.1, -0.05, -0.025, 0.0]
                    n23 = Multiply(x=w45, y=2) -> (x*y=w46:sgl[])
                    n24 = Select(t=w45, s=w44, f=w46) -> (s? t:f=w43:sgl[])
                  }
                }
                n25 = case shown="12" w35 {
                  tunnel: [string[] ["10 MS/s", "20 MS/s", "25 MS/s\n", "40 MS/s", "50 MS/s", "100 MS/s", "200 MS/s", "250 MS/s", "400 MS/s"] ("Strings []") string[] ["10 MS/s", "20 MS/s", "25 MS/s\n", "50 MS/s", "100 MS/s", "200 MS/s", "250 MS/s", "500 MS/s", "1 GS/s"] ("Strings []") string[] ["10 MS/s", "20 MS/s", "25 MS/s\n", "40 MS/s", "50 MS/s", "100 MS/s", "200 MS/s", "250 MS/s", "400 MS/s", "500 MS/s", "1 GS/s"] ("Strings []")] -> w34
                  tunnel: [string[] ["10 V", "5 V", "2 V", "1 V", "500 mV\n", "250 mV"] ("Strings []") string[] ["10 V", "4 V", "2 V", "1 V", "400 mV\n", "200 mV", "100 mV"] ("Strings []") string[] ["5 V", "2 V", "1 V", "500 mV", "200 mV", "100 mV\n", "50 mV"] ("Strings []")] -> _
                  frame 12 {
                  }
                  frame 1 {
                  }
                  frame 8, Default {
                  }
                }
                n26 = call "DAQ Assistant"("data"=bool[] [FALSE]) -> ()  [unwired: 3 in, 16 out]
                n27 = property on="Sampling Rate" class="Ring (strict)"("Strings []"=w34) -> ()  [unwired: 2 in, 2 out]
              }
              frame #1 {
                # "These are microseconds"
                n28 = global read "MotionGlobals.vi" "Additional dig delay (ms)"() -> (w82)
                n29 = global read "MotionGlobals.vi" "Digitizer delay\n (ms)"() -> (w80)
                n30 = global read "MotionGlobals.vi" "Offset delay (ms)"() -> (w83)
                n31 = global read "MotionGlobals.vi" "Samp Rate (Hz)"() -> (w68)
                n32 = expression code="x*1E-3"("Voltage Step Size (mVpp)") -> (w88:dbl)
                n33 = expression code="x*1E-3"("Start voltage (mVpp)") -> (w86:dbl)
                n34 = Unbundle By Name("RF data Out") -> ("rf points per line"=w92:u16)
                n35 = Compound Arithmetic op=ADD(w80, w82, w83) -> (w81:i32)
                n36 = Bundle("Samp Rate (Hz)"=w68, w81) -> (w79:cluster{"Samp Rate (Hz)":void, i32})  [unwired: 1 out]
                n37 = for {
                  N: "Num Freq Steps" -> [_]
                  tunnel: "Num Voltage Steps" -> [w115]
                  tunnel: w92 -> [w114]
                  tunnel: w91 -> [w113]
                  tunnel: w90 -> [w112]
                  tunnel: w88 -> [w111]
                  tunnel: w86 -> [w110]
                  tunnel: w85 -> [w109]
                  tunnel: w84 -> [w108]
                  tunnel: w79 -> [w107]
                  tunnel: "Vert Settings" -> [w95]
                  tunnel: w75 -> [w106]
                  tunnel: w74 -> [w105]
                  tunnel: w73 -> [w104]
                  tunnel: w72 -> [w103]
                  tunnel: "Freq Step Size (MHz)" -> [w101]
                  tunnel: "Start frequency (MHz)" -> [w100]
                  tunnel: w68 -> [w99]
                  tunnel: [w98] -> w55 mode=indexing
                  tunnel: [w97] -> w60 mode=indexing
                  tunnel: [w96] -> w56 mode=indexing
                  tunnel: [w93] -> w65 mode=indexing
                  tunnel: [w94] -> w57 mode=indexing
                  i -> [w102]
                  n38 = for {
                    N: w115 -> [_]
                    tunnel: w111 -> [w140]
                    tunnel: w110 -> [w139]
                    tunnel: w109 -> [w138]
                    tunnel: w114 -> [w137]
                    shift-right: [w136] -> _
                    shift-left: w95 -> [w135]
                    tunnel: w105 -> [w134]
                    tunnel: w112 -> [w133]
                    tunnel: w113 -> [w132]
                    tunnel: w108 -> [w131]
                    tunnel: w106 -> [w130]
                    tunnel: w107 -> [w129]
                    tunnel: w104 -> [w128]
                    tunnel: w103 -> [w127]
                    tunnel: w102 -> [w126]
                    tunnel: w101 -> [w125]
                    tunnel: w100 -> [w124]
                    tunnel: w99 -> [w123]
                    tunnel: [w122] -> w98 mode=indexing
                    tunnel: [w117] -> w97 mode=indexing
                    tunnel: [w121] -> w96 mode=indexing
                    tunnel: [w120] -> w93 mode=indexing
                    shift-right: [w119] -> _
                    shift-left: w95 -> [w118]
                    tunnel: [w116] -> w94 mode=indexing
                    i -> [w141]
                    n39 = stacked-sequence {
                      tunnel: w141 -> [w155 _ _]
                      tunnel: w140 -> [w154 _ _]
                      tunnel: w139 -> [w153 _ _]
                      tunnel: w138 -> [_ _ w181]
                      tunnel: w137 -> [_ _ w179]
                      tunnel: w135 -> [_ _ w172]
                      tunnel: [_ _ w180] -> w136
                      tunnel: w134 -> [w152 _ _]
                      tunnel: w133 -> [_ _ w178]
                      tunnel: w132 -> [_ _ w177]
                      tunnel: w131 -> [_ _ w176]
                      tunnel: w130 -> [_ _ w175]
                      tunnel: w129 -> [_ _ w174]
                      tunnel: w128 -> [w151 _ _]
                      tunnel: w127 -> [w150 _ _]
                      tunnel: w126 -> [w147 _ _]
                      tunnel: w125 -> [w146 _ _]
                      tunnel: w124 -> [w145 _ _]
                      tunnel: w123 -> [_ _ w173]
                      tunnel: [_ _ w167] -> w122
                      tunnel: [_ _ w169] -> w117
                      tunnel: [w142 _ _] -> w121
                      tunnel: [w144 _ _] -> w120
                      tunnel: [_ _ w171] -> w119
                      tunnel: w118 -> [_ _ w170]
                      tunnel: [_ _ w168] -> w116
                      frame #0 {
                        # "Change Frequency of HP 33250"
                        n40 = Multiply(x=w147, y=w146) -> (x*y=w149:dbl)
                        n41 = Add(x=w145, y=w149) -> (x+y=w142:dbl)
                        "current f" <- w142
                        n42 = Multiply(x=w154, y=w155) -> (x*y=w148:dbl)
                        n43 = Add(x=w153, y=w148) -> (x+y=w144:dbl)
                        "current V" <- w144
                        n44 = expression code="x*10**6"(w142) -> (w143:dbl)
                        n45 = case shown="1" w152 {
                          tunnel: w144 -> [w156 w165]
                          tunnel: w143 -> [w157 w163]
                          tunnel: w151 -> [_ w162]
                          tunnel: w150 -> [w161 _]
                          frame 0, Default {
                            w158 = u16 0 items=["Amplitude", "Frequency", "Offset"] ("Parameter (0: Amplitude)")
                            w159 = u16 1 items=["Amplitude", "Frequency", "Offset"] ("Parameter (0: Amplitude)")
                            n46 = call <instrlib>:"ag33xxx - Waveform Parameters.vi"("Value (1.00)"=w157, "Parameter (0: Amplitude)"=w159, "VISA session"=w161) -> ("dup VISA session"=w160:refnum<visa-resource-name>)  [unwired: 7 in, 1 out]
                            n47 = call <instrlib>:"ag33xxx - Waveform Parameters.vi"("Value (1.00)"=w156, "Parameter (0: Amplitude)"=w158, "VISA session"=w160) -> ()  [unwired: 7 in, 2 out]
                          }
                          frame 1 {
                            w164 = 1 items=["Sine"=1, "Square"=2, "Triangle"=3, "Ramp Up"=4, "Ramp Down"=5, "DC"=6, "Ramp"=1001, "Pulse"=1005, "Sync"=1002, "Gaussian"=1003, "Exponential"=1004, "Noise"=1006] ("waveform")
                            n48 = call <instrlib>:"ww128x Configure Standard Waveform.vi"("amplitude"=w165, "frequency"=w163, "waveform"=w164, "instrument handle"=w162) -> ()  [unwired: 4 in, 4 out]
                          }
                        }
                      }
                      frame #1 {
                        n49 = Wait (ms)(milliseconds to wait=500) -> ()  [unwired: 1 out]
                      }
                      frame #2 {
                        n50 = while {
                          tunnel: w181 -> [w208]
                          shift-right: [w207] -> w180
                          shift-left: w172 -> [w206]
                          tunnel: w179 -> [w205]
                          tunnel: w178 -> [w204]
                          tunnel: w177 -> [w203]
                          tunnel: w176 -> [w199]
                          tunnel: w175 -> [w198]
                          tunnel: w174 -> [w197]
                          tunnel: w173 -> [w196]
                          tunnel: [w189] -> w169
                          shift-right: [w191] -> w171
                          shift-left: w170 -> [w190]
                          tunnel: [w186] -> w168
                          tunnel: [w184] -> w167
                          i -> [w202]
                          stop <- w187 stop-if-true
                          n51 = stacked-sequence {
                            seq-local: [w212 _] -> [_ w287]
                            seq-local: [w211 _] -> [_ w288]
                            seq-local: [w218 _] -> [_ w286]
                            seq-local: [w219 _] -> [_ w285]
                            tunnel: w208 -> [w226 w282]
                            tunnel: [_ w293] -> w207
                            tunnel: w206 -> [_ w294]
                            tunnel: w205 -> [w225 _]
                            tunnel: w204 -> [_ w289]
                            tunnel: w203 -> [_ w283]
                            tunnel: [_ w297] -> w192
                            tunnel: w199 -> [w224 w292]
                            tunnel: w198 -> [w223 w284]
                            tunnel: w197 -> [w222 _]
                            tunnel: w196 -> [w220 _]
                            tunnel: [w219 _] -> w195
                            tunnel: [w218 _] -> w194
                            tunnel: [w212 _] -> w183
                            tunnel: [w211 _] -> w185
                            tunnel: [_ w296] -> w191
                            tunnel: w190 -> [_ w295]
                            tunnel: [w213 _] -> w186
                            frame #0 {
                              n52 = for {
                                N: "Average" -> [_]
                                tunnel: w226 -> [w246]
                                tunnel: w225 -> [w245]
                                tunnel: w224 -> [w244]
                                tunnel: w223 -> [w243]
                                tunnel: w222 -> [w242]
                                tunnel: w220 -> [w241]
                                tunnel: [w239] -> w217 mode=indexing
                                tunnel: [w238] -> w216 mode=indexing
                                tunnel: [w237] -> w215 mode=indexing
                                tunnel: [w236] -> w214 mode=indexing
                                tunnel: [w227] -> w213
                                n53 = case shown="1, Default" w244 {
                                tunnel: w246 -> [w255 _]
                                tunnel: w245 -> [w247 w263]
                                tunnel: [w253 w277] -> w234
                                tunnel: w243 -> [_ w275]
                                tunnel: w242 -> [w248 w269]
                                tunnel: [_ w262] -> w235
                                tunnel: [w247 w263] -> _
                                frame 0 {
                                w254 = 1
                                n54 = call <instrlib>:"Configure Memory Settings.vi"("Number of Samples (1000)"=w247, "Number of Segments (1)"=w254, "Instrument ID"=w255) -> ("error out"=w249:errorcluster, "dup Instrument ID"=w252:u32)  [unwired: 1 in, 2 out]
                                n55 = call "conSamp.vi"("error in"=w249, "Sampling"=w248, "InstrumentID"=w252) -> ("error out"=w250:errorcluster, "DUP ID"=w251:u32)
                                n56 = call <instrlib>:"Start Acquisition.vi"("error in (no error)"=w250, "Instrument ID"=w251) -> ("error out"=w259:errorcluster, "dup Instrument ID"=w260:u32)  [unwired: 2 in]
                                n57 = call <instrlib>:"Wait For End Of Acquisition.vi"("error in (no error)"=w259, "Timeout"=300, "Instrument ID"=w260) -> ("error out"=w257:errorcluster, "dup Instrument ID"=w258:u32)  [unwired: 3 out]
                                n58 = call "GetWaveform.vi"("Acq ID Out"=w258, "Read Mode"=enum32{"ADC", "Volts"}."Volts", "Num Samps"=w247, "Num Segs"=w254, "error in"=w257) -> ("first row"=w253:dbl[])  [unwired: 1 in, 9 out]
                                }
                                frame 1, Default {
                                n59 = property class="niScope"(reference=w275, "Min Number of Points"=w263, "Number of Records"=1) -> (reference out=w271:refnum<k15>, error out=w270:errorcluster)  [unwired: 1 in]
                                n60 = call "NI conSamp.vi"("error in"=w270, "Sampling"=w269, "InstrumentID"=w271) -> ("error out"=w272:errorcluster, "DUP ID"=w273:refnum<k15>)
                                n61 = call <instrlib>:"niScope Initiate Acquisition.vi"("instrument handle"=w273, "error in"=w272) -> ("instrument handle out"=w278:refnum<k15>, "error out"=w279:errorcluster)  [unwired: 12 out]
                                n62 = call-poly <instrlib>:"niScope Fetch (poly).vi"("timeout"=0.5, "error in"=w279, "channels"="0", "instrument handle"=w278) -> ("error out"=w266:errorcluster, "wfm"=w277:dbl[], "instrument handle out"=w264:refnum<k15>)  [unwired: 1 in, 4 out]
                                n63 = call-poly <instrlib>:"niScope Fetch (poly).vi"("timeout"=0.5, "error in"=w266, "channels"="1", "instrument handle"=w264) -> ("wfm"=w262:dbl[])  [unwired: 1 in, 6 out]
                                }
                                }
                                n64 = Multiply(x="Record Window (uS)", y=1e-06) -> (x*y=w230:dbl)
                                n65 = Multiply(x=w230, y=w241) -> (x*y=w240:dbl)
                                n66 = Array Size(array=w234) -> (size(s)=w233:i32)
                                n67 = Subtract(x=w233, y=w240) -> (x-y=w232:i32)
                                n68 = Array Subset(array=w235, length=w240) -> (w231:dbl[])  [unwired: 1 in]
                                "Ch 1" <- w231
                                n69 = Array Subset(array=w234, index=w232) -> (w227:dbl[])  [unwired: 1 in]
                                "Ch 0" <- w227
                                n70 = call-poly <vilib>:"Amplitude and Levels.vi"("signal in"=w231) -> ("low state level"=w238:dbl, "high state level"=w239:dbl)  [unwired: 7 in, 2 out]
                                n71 = call-poly <vilib>:"Amplitude and Levels.vi"("signal in"=w227) -> ("low state level"=w236:dbl, "high state level"=w237:dbl)  [unwired: 7 in, 2 out]
                              }
                              n72 = call-poly <vilib>:"Mean.vi"("X"=w216) -> ("mean"=w219:dbl)  [unwired: 1 out]
                              n73 = call-poly <vilib>:"Mean.vi"("X"=w217) -> ("mean"=w218:dbl)  [unwired: 1 out]
                              n74 = call-poly <vilib>:"Mean.vi"("X"=w215) -> ("mean"=w211:dbl)  [unwired: 1 out]
                              n75 = call-poly <vilib>:"Mean.vi"("X"=w214) -> ("mean"=w212:dbl)  [unwired: 1 out]
                            }
                            frame #1 {
                              n76 = call "Digitizer Voltage AutoScale.vi"("Card Type"=w283, "Vert Scale Lookup Table"=w289, "Main Digitizer"=w292, "NI Card"=w284, "Positive Peak"=w288, "Negitive Peak"=w287, "Channel"=0, "Acq Card ID"=w282, "Vert Settings In"=w294) -> ("Vert Settings Out"=w293:cluster{sgl, i32, "Coupling":u16}, "Success?"=w290:bool)
                              n77 = call "Digitizer Voltage AutoScale.vi"("Card Type"=w283, "Vert Scale Lookup Table"=w289, "Main Digitizer"=w292, "NI Card"=w284, "Positive Peak"=w286, "Negitive Peak"=w285, "Channel"=1, "Acq Card ID"=w282, "Vert Settings In"=w295) -> ("Vert Settings Out"=w296:cluster{sgl, i32, "Coupling":u16}, "Success?"=w291:bool)
                              n78 = And(x=w291, y=w290) -> (x .and. y?=w297:bool)
                            }
                          }
                          n79 = Equal?(x=10, y=w202) -> (x = y?=w200:bool)
                          n80 = Or(x=w192, y=w200) -> (x .or. y?=w187:bool)
                          n81 = case shown="False" "Inverting Hydrophone?" {
                            tunnel: w185 -> [_ w210]
                            tunnel: [w209 w210] -> w184
                            tunnel: w183 -> [w209 _]
                            frame False {
                            }
                            frame True {
                            }
                          }
                          n82 = Subtract(x=w194, y=w195) -> (x-y=w193:dbl)
                          n83 = Multiply(x="Attenuator", y=w193) -> (x*y=w189:dbl)
                        }
                      }
                    }
                  }
                }
                n84 = Multiply(x="Num Freq Steps", y="Num Voltage Steps") -> (x*y=w69:i32)
                n85 = call-poly <vilib>:"Plot Helper.vi"("z matrix"=w55) -> ("3D Plot lvclass Array out"=→"Ch 0":refnum<class "3D Plot Datatype.lvclass">[])  [unwired: 5 in, 5 out]
                n86 = Reshape Array(w56, w69) -> (w59:dbl[])
                n87 = Reshape Array(w65, w69) -> (w64:dbl[])
                n88 = Reshape Array(w55, w69) -> (w66:dbl[])
                n89 = Reshape Array(w60, w69) -> (w67:dbl[])
                n90 = call-poly <vilib>:"Plot Helper.vi"("z matrix"=w60) -> ("3D Plot lvclass Array out"=→"Ch 1":refnum<class "3D Plot Datatype.lvclass">[])  [unwired: 5 in, 5 out]
                n91 = Bundle(w59, w64, w66, w67) -> (w76:cluster{dbl[], dbl[], dbl[], dbl[]})  [unwired: 1 out]
              }
              frame #2 {
                # "turn off prf"
                # "FG drive\nvoltage matching (Vpp)\nvolt hydrop V\nPressure  neg MPa\nIntensity"
                n92 = call "DAQ Assistant2"("data"=bool[] [TRUE]) -> ()  [unwired: 3 in, 16 out]
                n93 = local write "Save Waveforms"("Auto Save Data?") -> ()
                n94 = local write "Save"("Auto Save Data?") -> ()
                "Data Array" <- w300
                "Waveform Array" <- w299
              }
            }
          }
          event "Save": Value Change {
            w313 = "\n"
            n95 = event-data() -> ()  [unwired: 7 out]
            n96 = local read "Transducer Info"() -> (w306:string)
            n97 = Get Date/Time String() -> (date string=w317:string, time string=w316:string)  [unwired: 3 in]
            n98 = local write "Save"(FALSE) -> ()
            n99 = Build Array(w317, w313, w316, w313, w306, w313, "Hydrophone Info", w313, "Amplifier Info", "Hydrophone Info", "Notes", "Hydrophone Info") -> (w312:string[])
            n100 = local read "File Path"() -> (w307:path)
            n101 = Concatenate Strings("Hydrophone Info", " " ("string"), w306, ".txt" ("element")) -> (w309:string)
            n102 = local read "Data Array"() -> (w323:cluster{dbl[], dbl[], dbl[], dbl[]})
            n103 = Build Path(base path=w307, name or relative path=w309) -> (appended path=w308:path)
            n104 = Build Array("Freq", "Voltage" ("element"), "Hydrophone Pk-Pk" ("element"), "Transducer Applied Voltage Pk-Pk" ("element")) -> (w328:string[])
            n105 = call-poly <vilib>:"Write To Spreadsheet File.vi"("1D data"=w312, "file path (dialog if empty)"=w308) -> ("new file path (Not A Path if cancelled)"=w315:path)  [unwired: 4 in, 2 out]
            n106 = Unbundle(w323) -> (w322:dbl[], w321:dbl[], w320:dbl[], w319:dbl[])
            n107 = Build Array(w322, w321, w320, w319) -> (w318:dbl[][])
            n108 = call-poly <vilib>:"Write To Spreadsheet File.vi"("append to file? (new file:F)"=TRUE, "1D data"=w328, "file path (dialog if empty)"=w315) -> ("new file path (Not A Path if cancelled)"=w330:path)  [unwired: 3 in, 2 out]
            n109 = call-poly <vilib>:"Write To Spreadsheet File.vi"("transpose? (no:F)"=TRUE, "append to file? (new file:F)"=TRUE, "2D data"=w318, "file path (dialog if empty)"=w330) -> ()  [unwired: 2 in, 3 out]
          }
          event "Save Waveforms": Value Change {
            w334 = "\n"
            n110 = event-data() -> ()  [unwired: 7 out]
            n111 = local read "Hydrophone Info"() -> (w337:string)
            n112 = local read "Transducer Info"() -> (w336:string)
            n113 = global read "MotionGlobals.vi" "Samp Rate (Hz)"() -> (w343)
            n114 = local read "Amplifier Info"() -> (w332:string)
            n115 = local read "File Path"() -> (w339:path)
            n116 = local read "Notes"() -> (w333:string)
            n117 = Concatenate Strings(w337, " " ("string"), w336, " Waveforms.xls" ("element")) -> (w340:string)
            n118 = Number To Decimal String(number=w343) -> (decimal integer string=w350:string)  [unwired: 1 in]
            n119 = Get Date/Time String() -> (date string=w356:string, time string=w355:string)  [unwired: 3 in]
            n120 = Build Path(base path=w339, name or relative path=w340) -> (appended path=w338:path)
            n121 = Build Array(w356, w334, w355, w334, w336, w334, w337, w334, w332, w334, w333, w334, "Sampling Rate (Hz): " ("element"), w350) -> (w352:string[])
            n122 = local read "Data Array"() -> (w357:cluster{dbl[], dbl[], dbl[], dbl[]})
            n123 = local read "Waveform Array"() -> (w349:dbl[][][])
            n124 = local write "Save Waveforms"(FALSE) -> ()
            n125 = Build Array("Freq", "Voltage" ("element"), "Data" ("element")) -> (w360:string[])
            n126 = call-poly <vilib>:"Write To Spreadsheet File.vi"("1D data"=w352, "file path (dialog if empty)"=w338) -> ("new file path (Not A Path if cancelled)"=w354:path)  [unwired: 4 in, 2 out]
            n127 = Unbundle(w357) -> (w347:dbl[], w346:dbl[])  [unwired: 2 out]
            n128 = call-poly <vilib>:"Write To Spreadsheet File.vi"("append to file? (new file:F)"=TRUE, "1D data"=w360, "file path (dialog if empty)"=w354) -> ("new file path (Not A Path if cancelled)"=w345:path)  [unwired: 3 in, 2 out]
            n129 = for {
              tunnel: w346 -> [w366]
              tunnel: w347 -> [w367]
              tunnel: w349 -> [w369] mode=indexing
              shift-right: [w365] -> _
              shift-left: 0.0 -> [w364]
              tunnel: w345 -> [w363]
              i -> [w368]
              n130 = for {
                tunnel: w369 -> [w378] mode=indexing
                tunnel: w367 -> [w377]
                tunnel: w366 -> [w376]
                shift-right: [w372] -> w365
                shift-left: w364 -> [w371]
                tunnel: [w370] -> w362 mode=indexing
                i -> [w373]
                n131 = Index Array(array=w377, index=w371) -> (element=w375:dbl)
                n132 = Index Array(array=w376, index=w371) -> (element=w374:dbl)
                n133 = Build Array (concatenate)(w375, w374, w378) -> (w370:dbl[])
                n134 = Increment(x=w371) -> (x+1=w372:dbl)
                "Numeric" <- w373
              }
              n135 = call-poly <vilib>:"Write To Spreadsheet File.vi"("append to file? (new file:F)"=TRUE, "2D data"=w362, "file path (dialog if empty)"=w363) -> ()  [unwired: 3 in, 3 out]
              "Numeric 2" <- w368
            }
          }
          event "Set up Digi": Value Change {
            n136 = event-data() -> ()  [unwired: 2 out]
            n137 = call "SetUpDigi.vi"("Motion Settings Out"="Motion Bd ID", "Therapy (T)"=FALSE, 8:TRUE ("33250(T)/33120(F)")) -> ("RF data Sampling Out"=w383:T3, "Vert Settings"=w384:cluster{dbl, dbl, "Coupling":u16})  [unwired: 4 in, 3 out]
            n138 = local write "Vert Settings"(w384) -> ()
            n139 = local write "RF data Out"(w383) -> ()
            n140 = local write "Set up Digi"(FALSE) -> ()
          }
        }
      }
    }
    frame #2 {
      n141 = case shown="0, Default" w387 {
        tunnel: w386 -> [_ w390]
        tunnel: w385 -> [w389 _]
        frame 0, Default {
          n142 = call <instrlib>:"ag33xxx - Close.vi"("VISA session"=w389) -> ()  [unwired: 10 in, 1 out]
        }
        frame 1 {
          n143 = call <instrlib>:"ww128x Close.vi"("instrument handle"=w390) -> ()  [unwired: 1 in, 10 out]
        }
      }
      n144 = call <instrlib>:"niScope Close.vi"("instrument handle"=w388) -> ()  [unwired: 1 in, 14 out]
    }
  }
  n145 = local write "Save Waveforms"(w1) -> ()
  n146 = local write "Save"(w1) -> ()
  n147 = local write "Transducer Info"("Transducer Info") -> ()
